vi "MainPannelFastEnabled.vi"() -> ()   [LabVIEW 2020]
uses:
  Digi/Controls/DigiMachineStates.ctl
  Digi/Digitizer_StatesMain.ctl
  <vilib>/userdefined/High Color/nirio_resource_hc.ctl
  Stage/New/StageOptions.ctl
  FileStore/Data Save State.ctl
  Gen/Generator_States.ctl
  <vilib>/Heliosphere Research LLC/Advanced Plotting Toolkit/properties/Colormap_Map.ctl
  <vilib>/Native 3D Graph/xcontrol/3DPC_SurfacePlot.xctl
  WaveClusterPacket.ctl
  ThorLabs/SubViForControl/Z Axis States.ctl
  <vilib>/UPVI/lvhdf5/library.llb/HDF5 Ref.ctl
  ImageCluster.ctl
  ThorLabs/SubViForControl/Thor_KCubeServoDCRef.ctl
  ThorLabs/SubViForControl/Thor_DeviceRef.ctl
  LongShotStates.ctl
  <vilib>/Platform/TimedLoop/XDataNode/timing_clust.ctl
  <vilib>/Platform/TimedLoop/XDataNode/nitl_modes.ctl
  <vilib>/Platform/TimedLoop/XDataNode/wakeup.ctl
  Stage/New/SettingCtrlOptions.ctl
  Stage/New/PosCtrlOptions.ctl
  Digi/Controls/FPGA VI Reference.ctl
  <extravilib>/ChannelInstances/Tag-bool/Read With Abort.vi
  <extravilib>/ChannelInstances/Tag-a[.](dbl)/Read With Abort.vi
  <extravilib>/ChannelInstances/Tag-a[.](dbl)/Write With Abort.vi
  <extravilib>/ChannelInstances/Tag-bool/Write With Abort.vi
  <extravilib>/ChannelInstances/Tag-bool/Instantiate.vi
  <extravilib>/ChannelInstances/Tag-bool/EndpointRead.vi
  <vilib>/FPGAPlugInAG/PXIe-7962R/niLvFpga_Open_PXIe-7962R.vi
  <vilib>/rvi/interface/common/dynamic/niFpgaDynamicAddResources.vi
  <vilib>/FPGAPlugInAG/Dynamic/niLvFpga_Close_Dynamic.vi
  <extravilib>/ChannelInstances/Tag-bool/Endpoint.vi
  <extravilib>/ChannelInstances/Tag-a[.](dbl)/Instantiate.vi
  <extravilib>/ChannelInstances/Tag-a[.](dbl)/EndpointRead.vi
  <extravilib>/ChannelInstances/Tag-a[.](dbl)/Endpoint.vi
  <vilib>/Platform/TimedLoop/XDataNode/XDataNode.xnode
  <vilib>/rvi/interface/nirviOpenFPGA/nirviOpenFPGA.xnode
  FPGA Bitfiles/DigitizerFPGACode(Fully_Functional)_v3.lvbitx
  <vilib>/rvi/interface/nirviCloseFPGA/nirviCloseFPGA.xnode
  <instrlib>/_niInstr/Basic Elements/v1/FPGA/niInstr Basic Elements v1 FPGA.lvlib
  <vilib>/Platform/TimedLoop/XDataNode/XDNodeRunTimeDep.lvlib
  Stage/libximc.lvlib
  <extravilib>/ChannelInstances/Tag-bool.lvlib
  <extravilib>/ChannelInstances/Tag-a[.](dbl).lvlib
  E:/Norway Project/All Hardware/New Microscope/LabVIEW/ThorLabs/Thorlabs.MotionControl.Controls.dll
  ThorLabs/Thorlabs.MotionControl.Controls.dll
  E:/Norway Project/All Hardware/New Microscope/LabVIEW/ThorLabs/ThorLabs.MotionControl.KCube.DCServoCLI.dll
  ThorLabs/ThorLabs.MotionControl.KCube.DCServoCLI.dll
  <vilib>/Heliosphere Research LLC/Advanced Plotting Toolkit/Advanced Plotting Toolkit.lvlib
panel:
  out "ProgressBar\nLongShot":u8(slide) scale=0.0..100.0
  in  "Long Shot Time (us)":dbl
  in  "LongShot":bool
  out "At Limit":bool
  out "Z Moving?":bool
  in  "Z_Speed (mm/s)":dbl=0.5 caption="Speed (mm/s)" min=0.0 max=10.0 step=0.1
  out "Z Open?":bool
  out "Z (mm)":dbl format="%#.3g"
  in  "Z_Stop":bool
  in  "Z_MoveDown":bool
  in  "Z_Move Up":bool
  in  "Z Step (mm)":dbl=0.1 min=0.0 max=50.0 step=0.01
  out "RemainingTimeString":string
  out "ProgressBar":u8(slide) scale=0.0..100.0
  out "Image Display":dbl[][](graph)
  in  "Colormap Selector":T1(ring)=enum."gray"
  in  "Save Img":bool
  in  "LogMode":bool
  in  "Start Digitizer UI Bttn":bool
  out "Max Index (s)":dbl format="%#_3p"
  out "Max Val (V)":dbl format="%#_3p"
  in  "Delay_Scroll_Range":dbl=2.0 caption="Range"
  in  "FineDelayControl":dbl(slide)=1.0 step=0.1 scale=19.5..23.5
  in  "Amplitude Range":cluster{"Slider 1":dbl, "Slider 1":dbl}(slide)={"Slider 1"=1.0, "Slider 1"=1.6299559471365639} scale=-2.5..2.5
  in  "Pause Triggger":bool caption="Pause"
  in  "Delay(us)":sgl min=0 step=0.1 format="%#_4p"
  in  "Time Division":u8(slide)=1 max=2 step=1 scale=0.0..2.0
  in  "Amplitude \nAveraging":u16(slide)=1 caption="Amplitude Averaging" scale=0.0..7.0 scale format="%#.2g"
  in  "Record Size":u16=1024
  in  "RIO Resource":T2="PXI1Slot2"
  out "Configured?":bool
  out "TIS Configured?":bool
  out "Range (Vpp)":dbl=1.3
  out "Digitizer On":bool
  out "Waveform [LIVE]":cluster{"Start Time":dbl, dbl, ext[]}(graph)
  in  "TriggerDigi":bool
  in  "Scanning":bool
  in  "Single Shot":bool
  in  "LIVE":bool
  in  "Transducer Freq (Hz)":u64
  in  "Temperature (C)":dbl
  in  "Remarks":string
  in  "Immersion Medium":string
  in  "EXIT APP":bool
  in  "Save to File":bool=TRUE caption="Checkbox"
  out "No Trig Miss":bool
  in  "FileName":string="testing"
  in  "File Store Directory":path=path "C:/Prakhar/ScratchStart/Labview16/TrashTest"
  out "File Open?":bool
  out "X Step Size (R)":sgl format="%#_2g"
  out "Y Step Size (R)":sgl format="%#_2g"
  out "Scan Time (Approx.)":string
  out "Total Pixels":u64
  out "Moving?":bool
  out "Stage Position":cluster{sgl[], sgl[]}(graph) caption="XY Graph - Dark"
  in  "X Position Abs":dbl caption="X Position"
  in  "Y Position Abs":dbl caption="Y Position"
  out "Line Count":u64=6 caption="Y Pixels"
  out "Pixel Count":u64=6 caption="X Pixels"
  in  "X Start":sgl
  in  "X End":sgl=10.0
  in  "Y Start":sgl
  in  "Y End":sgl=8.0
  in  "Y Step Size":sgl=0.5
  in  "X Step Size":sgl=0.5
  in  "Scan Mode":enum16{"Raster", "Serpentine"}(ring)
  in  "Speed Control (mm/s)":sgl(slide)=4.0 min=0.1 scale=0.1..5.0
  in  "AbsMove":bool
  in  "Outline":bool
  in  "Start Stage":bool
  in  "Stop Motion":bool
  in  "Zero":bool
  in  "Right":bool
  in  "Left":bool
  in  "Move to Start":bool
  in  "Down":bool
  in  "Up":bool
  out "X Position":dbl format="%#.3g"
  out "Y Position":dbl format="%#.3g"
  in  "Move Step":dbl=1.0
  in  "Stop Stage":bool
  out "Controller Open?":bool
  in  "Developer Options Control":T3(tab)
  in  "Stop Gen App":bool
  out "Gen State":T4
  out "Error Out Gen":errorcluster
  in  "Send vi Trig":bool
  out "Gain":dbl
  out "Offset Factor":dbl
  out "Amplitudes":dbl[](array[numeric]) format="%.2f"
  out "Sampling Frequency (Hz)":u64
  out "Waves per Pixel":u32
  in  "Ext/nViTrig":bool=TRUE
  in  "Machine Mode":T5(ring)=enum."Normal"
  in  "Stop Stage App":bool
  out "Error Out Stage":errorcluster
  in  "Next Coordinate Index":i32
  in  "EdgePt/nPixelMap":bool=TRUE
  out "Coordinate Array":sgl[][](array[numeric])
  out "Step Sizes":sgl[](array[numeric])
  out "Peripheral Coordis":sgl[][](array[numeric])=[[0.0, 0.0], [1.8, 0.0], [3.6, 0.0], [5.3999996, 0.0], [7.2, 0.0], [9.0, 0.0], [9.0, 2.0], [7.2, 2.0], [5.3999996, 2.0], [3.6, 2.0], [1.8, 2.0], [0.0, 2.0], [0.0, 4.0], [1.8, 4.0], [3.6, 4.0], [5.3999996, 4.0], [7.2, 4.0], [9.0, 4.0], [9.0, 6.0], [7.2, 6.0], [5.3999996, 6.0], [3.6, 6.0], [1.8, 6.0], [0.0, 6.0], [0.0, 8.0], [1.8, 8.0], [3.6, 8.0], [5.3999996, 8.0], [7.2, 8.0], [9.0, 8.0], [9.0, 10.0], [7.2, 10.0], [5.3999996, 10.0], [3.6, 10.0], [1.8, 10.0], [0.0, 10.0]]
  in  "Correction Table Path (Hidden)":path
  out "Serial nos":u32[](array[numeric])
  out "Calibration":cluster{dbl, "MicrostepMode":u32}[](array[cluster])
  out "IDs":i32[](array[numeric])
  in  "X Max Stage":dbl=220.0 format="%#_13g"
  in  "Y Maximum":dbl=220.0
  out "Stage Status":T6
  out "Z Axis State":T7
  out "Wave Count Zero":bool
  in  "CountReset":bool
  in  "Trigger Digi Single":bool
  in  "Start Digi":bool
  in  "Stop Digi App":bool caption="Stop Digi \nApplication"
  in  "Digi Machine Mode":T8=enum."Single Shot Mode"
  out "Waves Count":u64
  in  "Imaging":bool
  out "Digi State":T9
  out "nDigiLoopRunning":bool
  out "error out Digi":errorcluster
  out "Wave out packet":T10
  out "Error Out FileIO":errorcluster
  in  "Done Recording":bool
  in  "Record Data":bool
  in  "Open File":bool
  in  "Stop File App":bool
  out "FileStore State":T11
  out "Scan Running":bool=TRUE
  out "Scan Complete":bool=TRUE
  out "AmplitudeArray":dbl[](array[numeric])
  out "IndexArray":dbl[](array[numeric])
  in  "Map":T12
  in  "ColorBar":bool
  in  "Axis":bool
  out "Scanned Image":picture
  out "Topography Plot":refnum<class "Base Datatype.lvclass">[](xcontrol)
  out "LongShotRunTimes":u32=6
  out "FilenameSimeStamped":string
  out "FileDirectoryFinal":path
  out "total time (sec)":sgl
  in  "Generator  Port":refnum<k15>="PXI1Slot3"
  out "Actual Sample Rate":dbl format="%#_6p"
  in  "Use Default Wave Settings":bool=TRUE caption="Checkbox"
  in  "Start Gen":bool
  in  "stop Gen":bool
  out "Generator On":bool
  out "Input Waveform":dbl[](graph)
  # "SAVE ALL CONFIGS TO FILE AND LOAD IT"
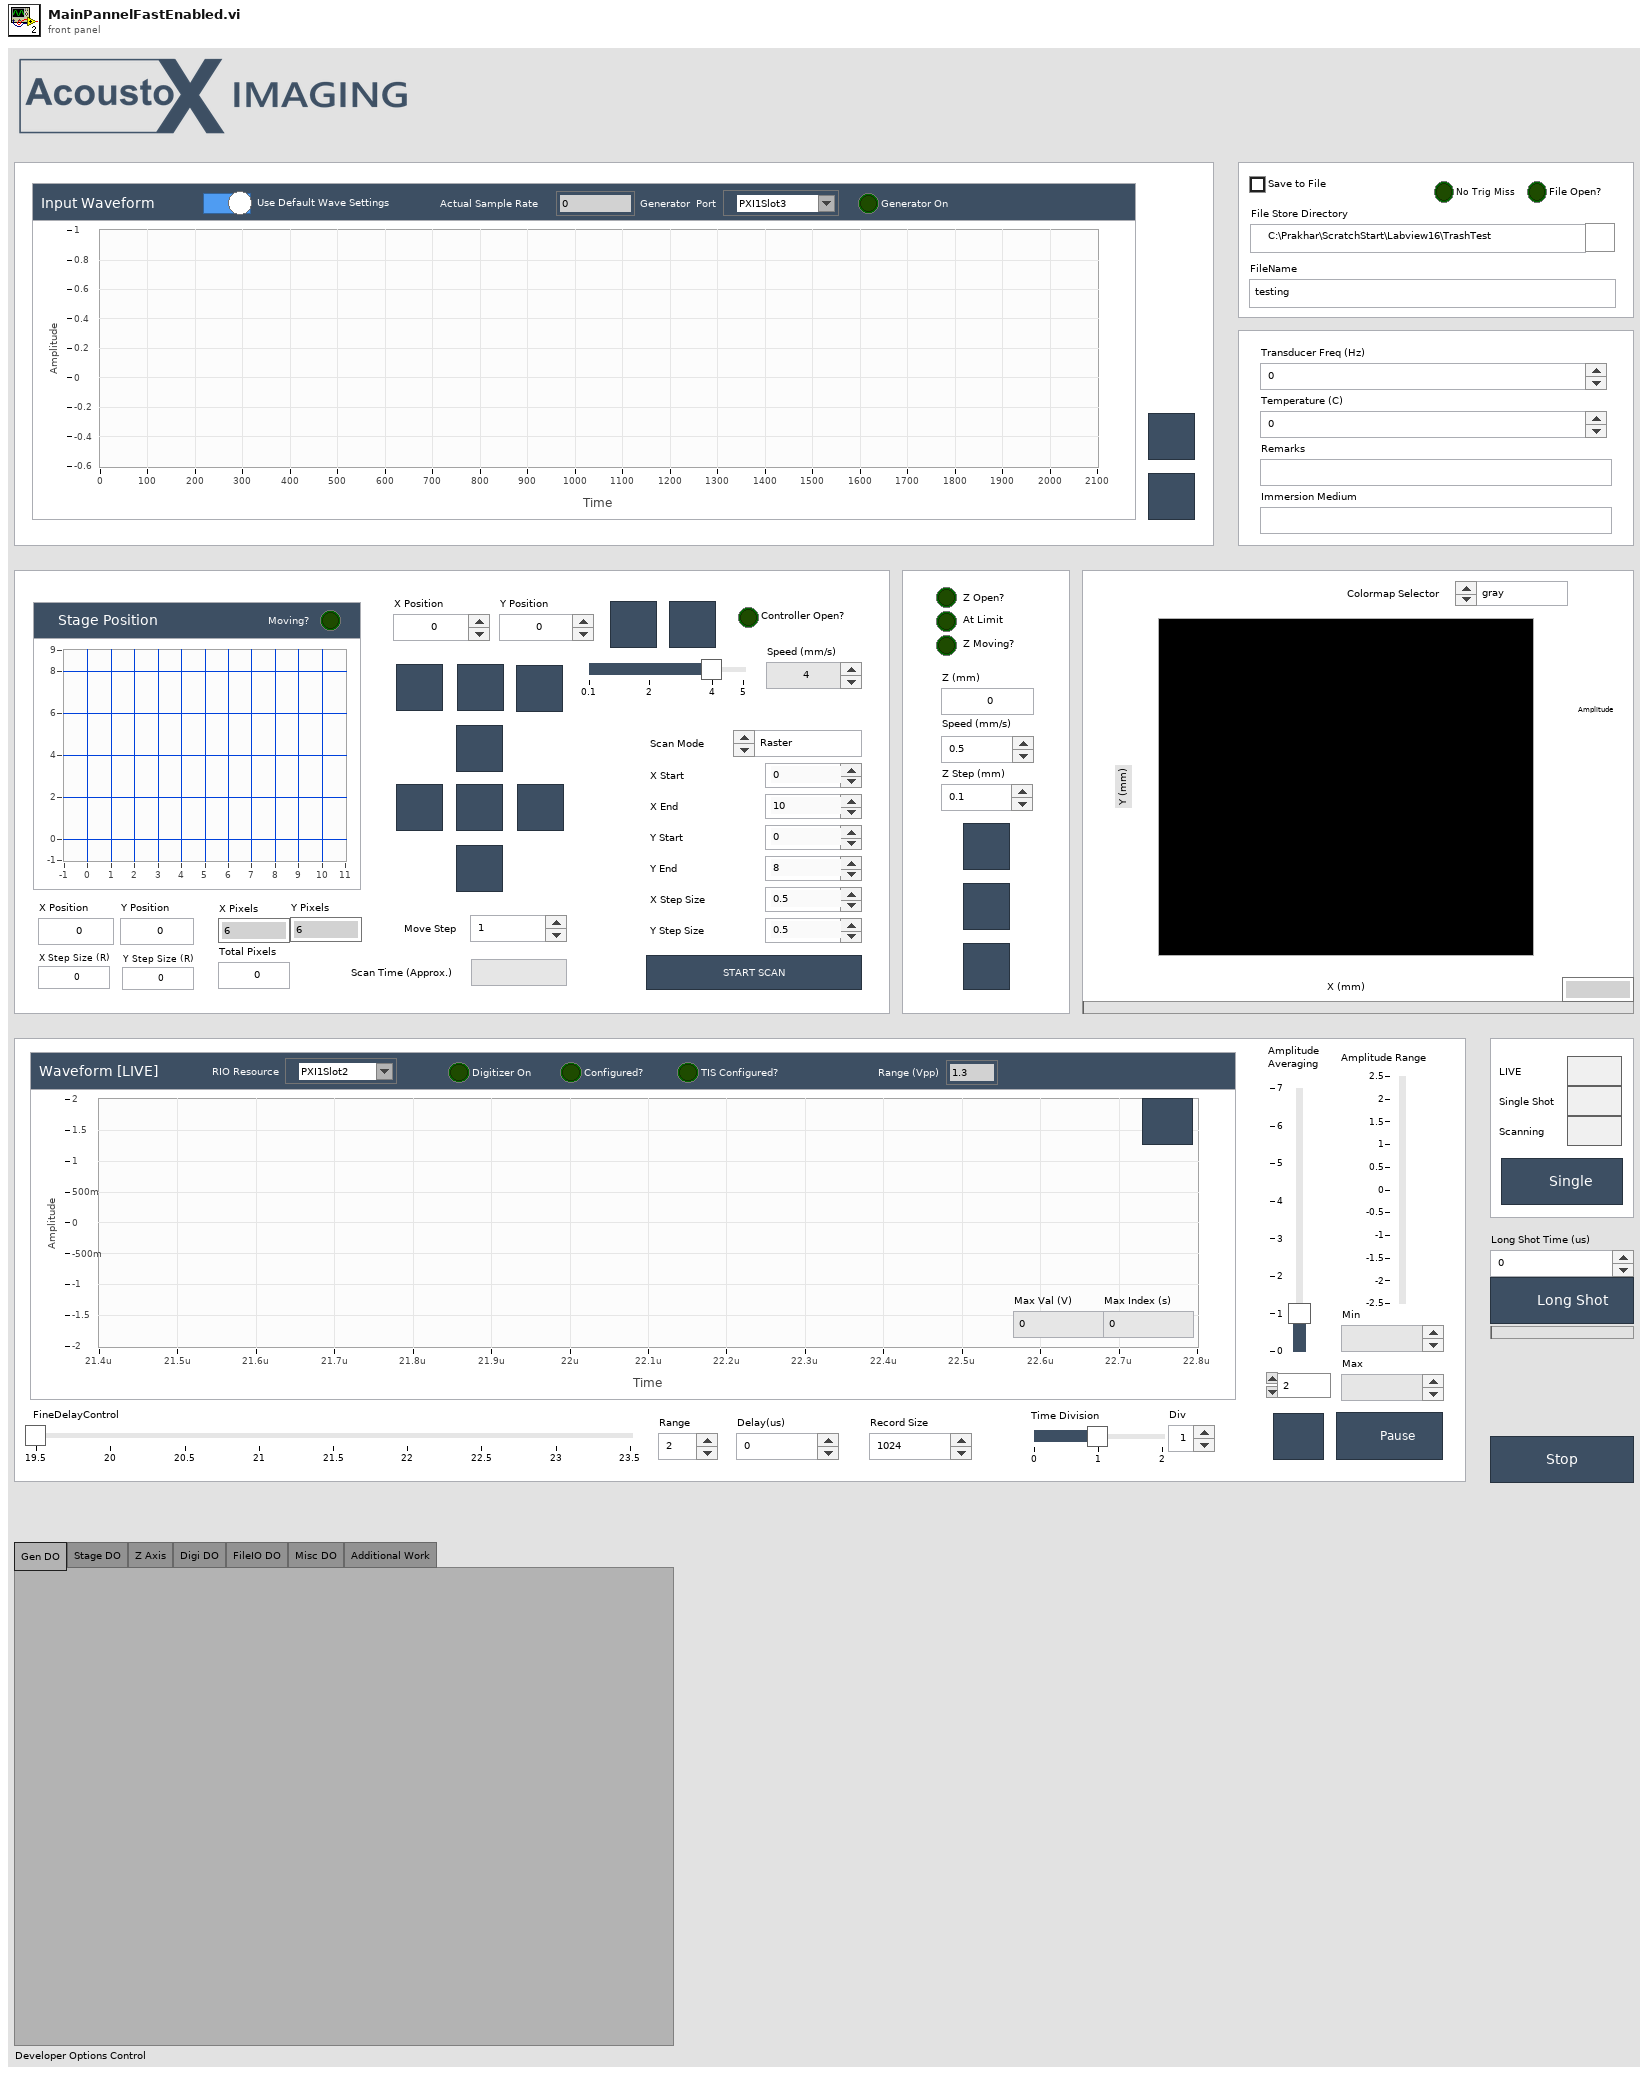
[diagram p1: front panel]
types:
  T1 = enum16{"fire", "rainbow", "gray", "inverse gray", "ice", "original"}
  T2 = typedef "nirio_resource_hc.ctl" = tag
  T3 = enum32{"Gen DO", "Stage DO", "Z Axis", "Digi DO", "FileIO DO", "Misc DO", "Additional Work"}
  T4 = typedef "Generator_States.ctl" = enum16{"Idle", "GenerateWaveArray", "InitGen", "SendVITrig", "CloseGen", "CloseApp"}
  T5 = enum16{"Scanning Mode", "Perimeter Mode", "Normal"}
  T6 = typedef "StageOptions.ctl" = enum16{"Idle", "Init", "Set Speed", "GenerateMotionPoints", "Scan_Start", "Scan_MoveNext", "Scan_SyncSet", "Scan_Get Pos", "Scan_Complete", "Cmd_MoveAbs", "Cmd_CloseControllers", "Cmd_MoveUp", "Cmd_MoveDown", "Cmd_MoveLeft", "Cmd_MoveRight", "Cmd_MoveStart", "Cmd_MoveZero", "Cmd_GetPos", "Cmd_Stop", "Sync_On", "Sync_Off", "Stop Motion", "CloseApplication"}
  T7 = typedef "Z Axis States.ctl" = enum16{"Idle", "Init", "cmd_MoveUp Rel", "cmd_MoveDown Rel", "cmd_GetPos", "cmd_SetVel", "cmd_stop", "Close Z"}
  T8 = typedef "DigiMachineStates.ctl" = enum16{"Scanning Mode", "Live Mode", "Single Shot Mode", "Idle Mode"}
  T9 = typedef "Digitizer_StatesMain.ctl" = enum16{"Idle", "Init", "SetParam", "VITrig", "Read", "CloseDigi", "CloseApp"}
  T10 = typedef "WaveClusterPacket.ctl" = cluster{"Wave Count":u64, "Wave":i16[]}
  T11 = typedef "Data Save State.ctl" = enum16{"Idle", "Open File", "Write Attributes", "Append Data", "Close File", "Close App"}
  T12 = typedef "Advanced Plotting Toolkit.lvlib/Colormap_Map.ctl" = enum16{"Automatic", "Rainbow", "Hot and Cold", "White-Black", "White-Blue", "White-Green", "White-Red", "Fire", "Water", "Earth", "Air", "Pastel", "Banded", "Stepped"}
  T13 = typedef "LongShotStates.ctl" = enum16{"Idle", "Start Gen", "Set Digi Mode", "Clear Wave Count", "Set Initial Param", "Set Param", "Take Shot", "UpdateParam", "Show Data"}
  T14 = typedef "Thor_DeviceRef.ctl" = refnum<k24>
  T15 = typedef "Thor_KCubeServoDCRef.ctl" = refnum<k24>
  T16 = typedef "ImageCluster.ctl" = cluster{"Wave Count":u64, "Amplitude":i16, "Index":u16}
  T17 = typedef "HDF5 Ref.ctl" = refnum<k1>
  T18 = typedef "XDNodeRunTimeDep.lvlib/timing_clust.ctl" = cluster{"Expected End [f-1]":u64, "Actual End [f-1]":u64, "Finished Late? [f-1]":bool, "Expected End [i-1]":u64, "Actual End [i-1]":u64, "Finished Late? [i-1]":bool, "Expected Start [i]":u64, "Actual Start [i]":u64, "Expected Start [f]":u64, "Actual Start [f]":u64, "Source Name":string, "Structure Name":string, "Period":i64, "Deadline":i64, "Offset":i64, "Start":i64, "Priority":i32, "Timeout":i32, "Mode":T19, "Wakeup Reason":T20, "Error":errorcluster, "Source Type":string, "Secondary Source Type":string, "Global End Time":u64, "Global Start Time":u64, "Frame Duration":u64, "Iteration Duration":u64, "Assigned CPU":i32, "I/O Scan Engine Mode":u32}
  T19 = typedef "XDNodeRunTimeDep.lvlib/nitl_modes.ctl" = enum32{"No Change", "Process missed periods, maintain original phase", "Discard missed periods, maintain original phase", "Process missed periods, ignore original phase", "Discard missed periods, ignore original phase"}
  T20 = typedef "XDNodeRunTimeDep.lvlib/wakeup.ctl" = enum32{"Normal", "Aborted", "Asynchronous wakeup", "Timing source error", "Timed loop error", "Timeout"}
  T21 = typedef "SettingCtrlOptions.ctl" = enum16{"Set X", "Set Y", "Set X and Y", "Get Settings", "None"}
  T22 = typedef "PosCtrlOptions.ctl" = enum16{"Move X", "Move Y", "Both X and Y", "Read Pos", "None"}
  T23 = typedef "Tag-a[.](dbl).lvlib/))Channel.ctl" = refnum<queue>
  T24 = typedef "FPGA VI Reference.ctl" = refnum<k20>
  T25 = typedef "imagedata.ctl" = cluster{"image type":i32, "image depth":i32, "image":u8[], "mask":u8[], "colors":u32[], "Rectangle":cluster{"left":i16, "top":i16, "right":i16, "bottom":i16}}
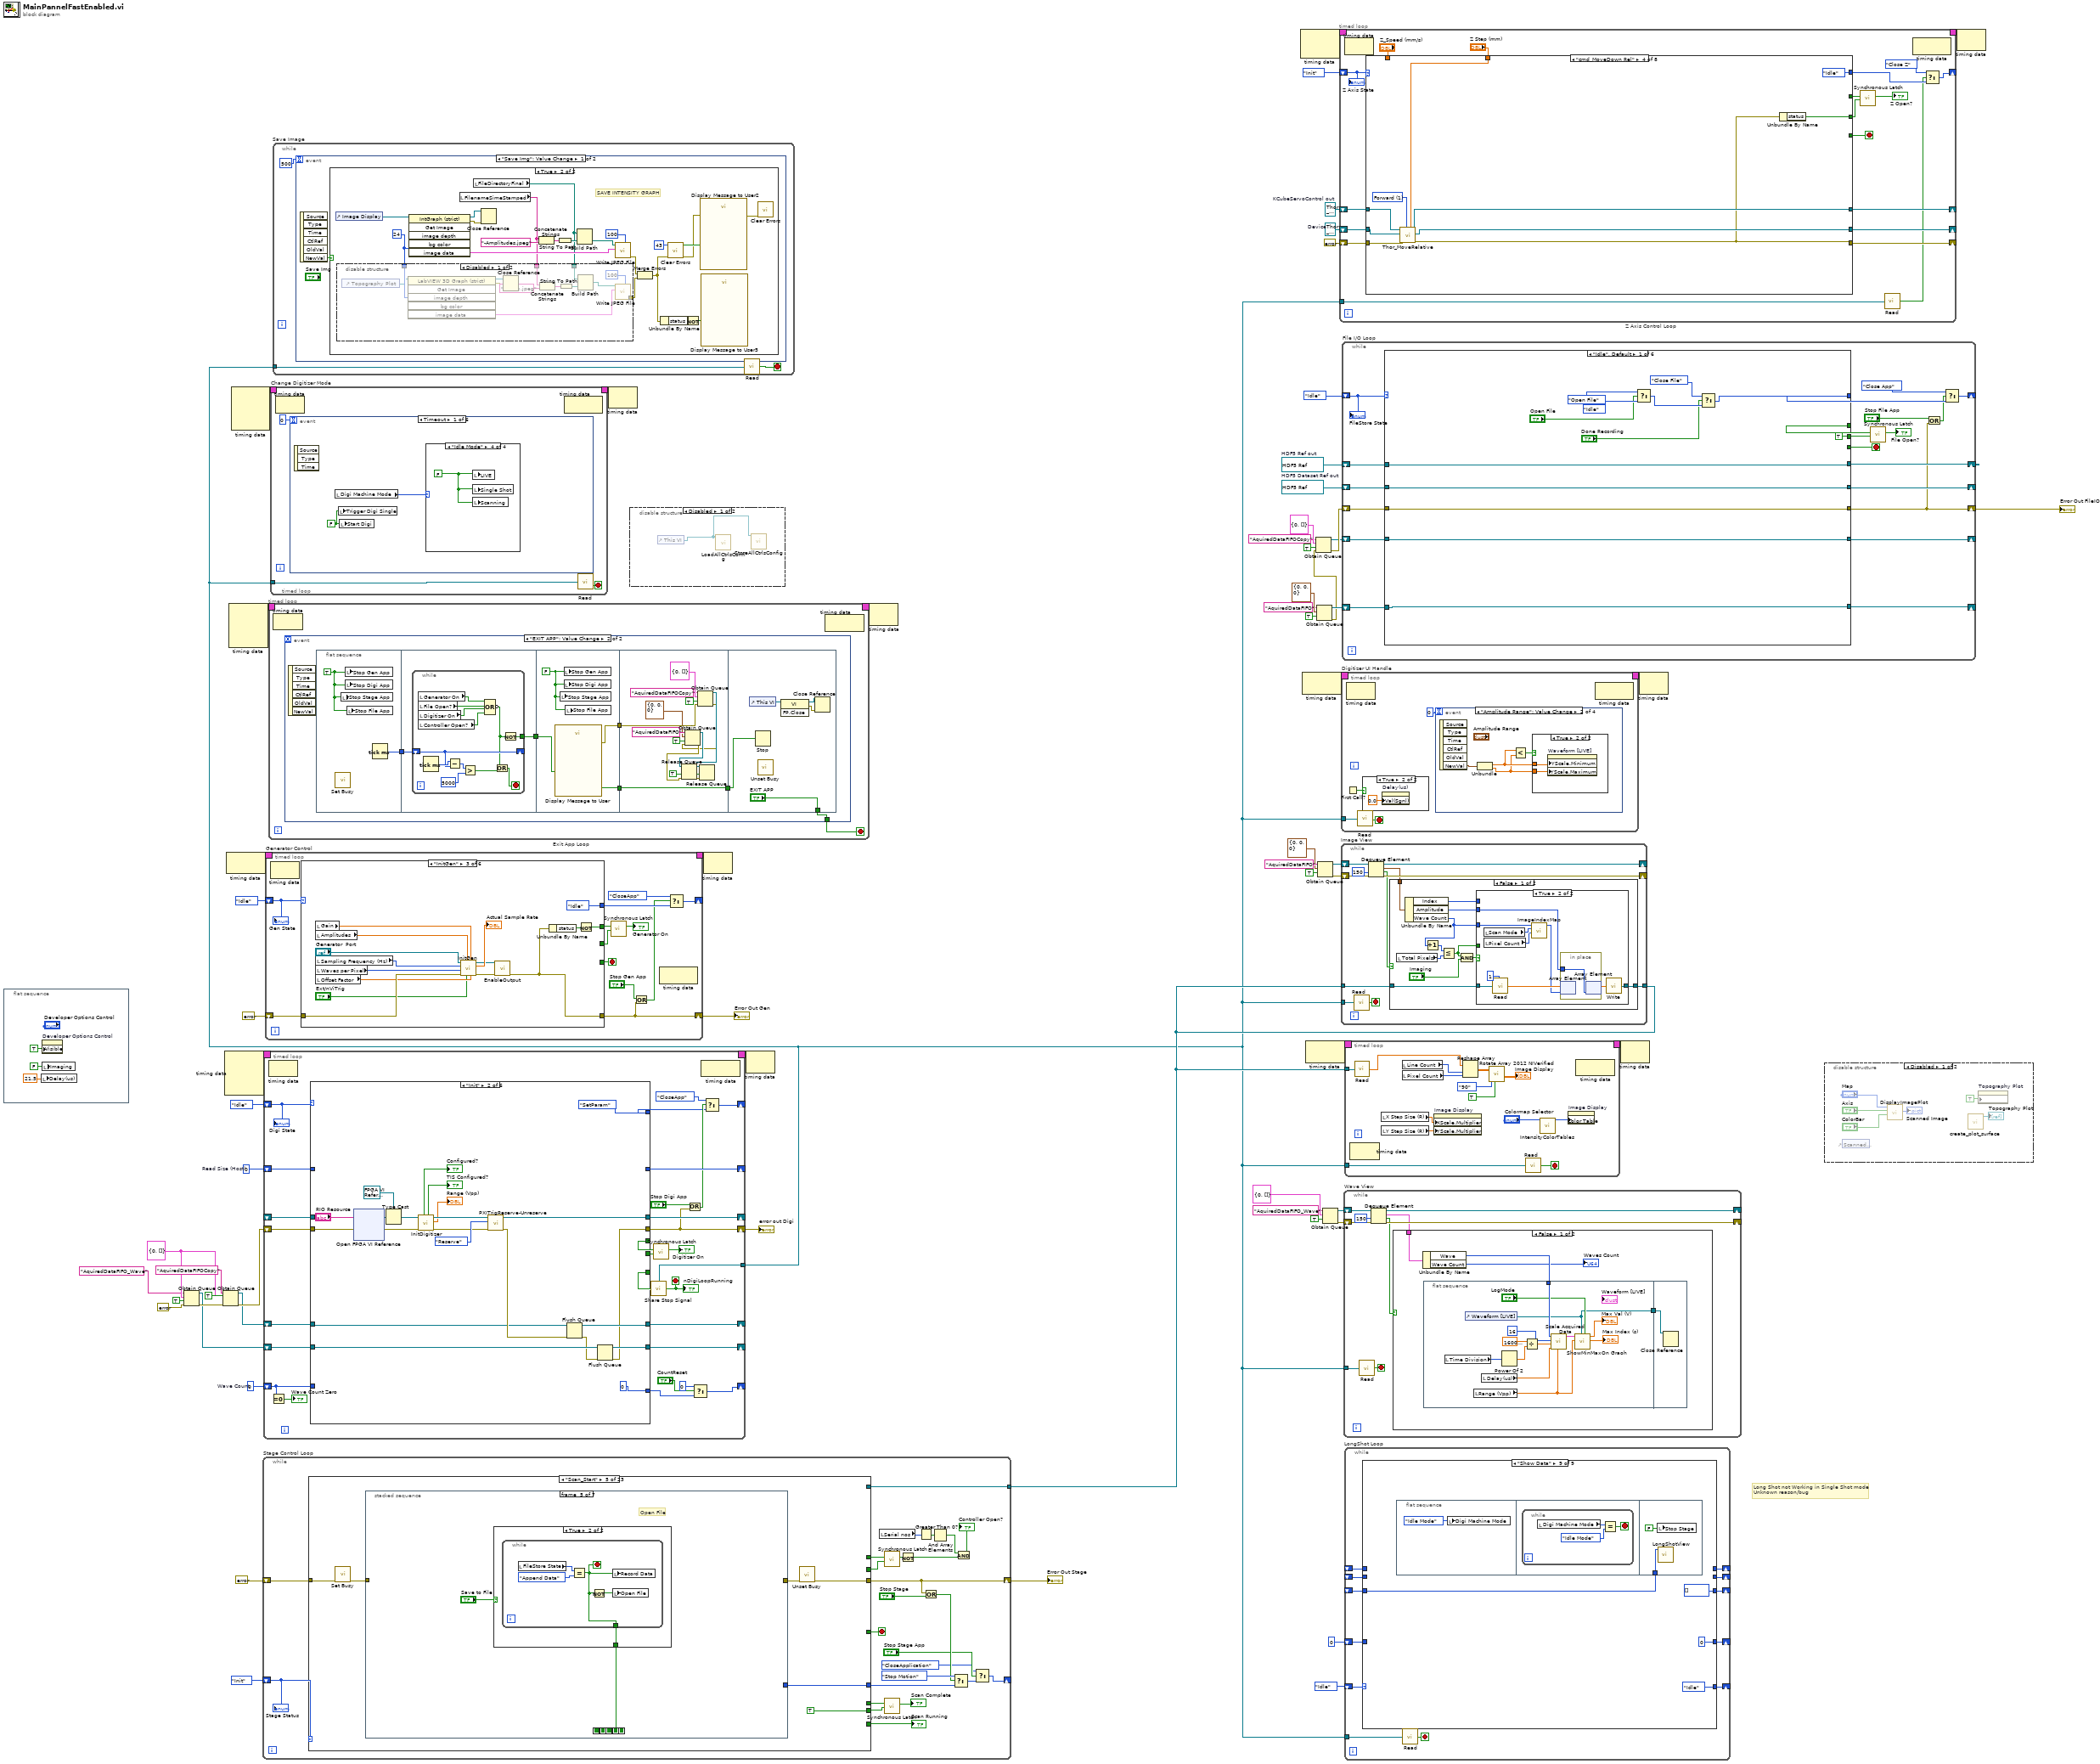
[diagram p0: block diagram]
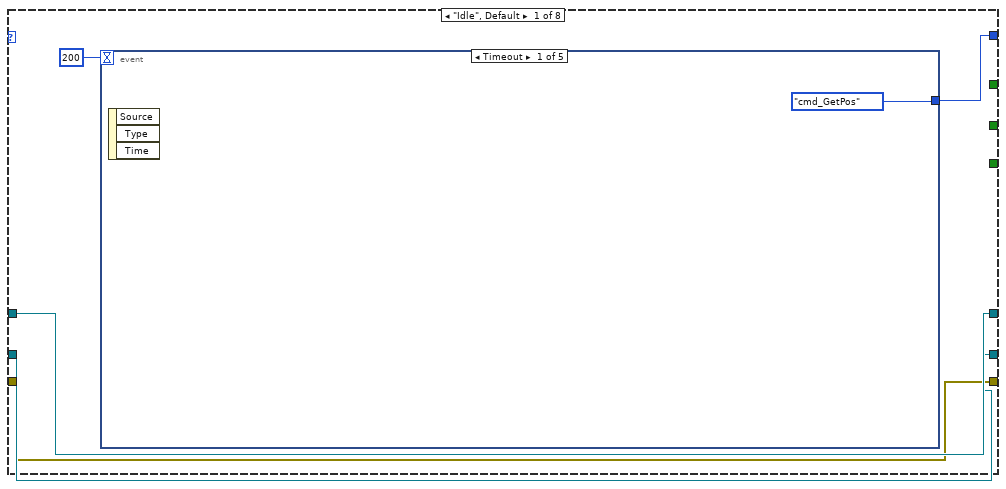
[diagram p2: hidden frame]
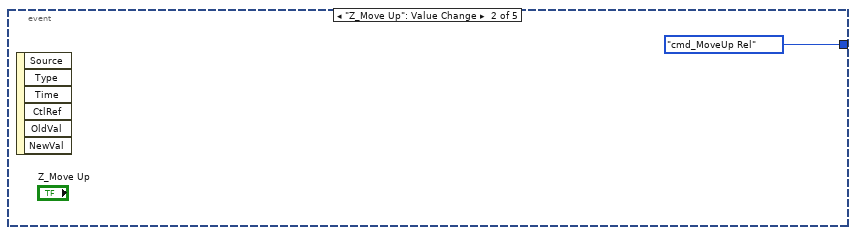
[diagram p3: hidden frame]
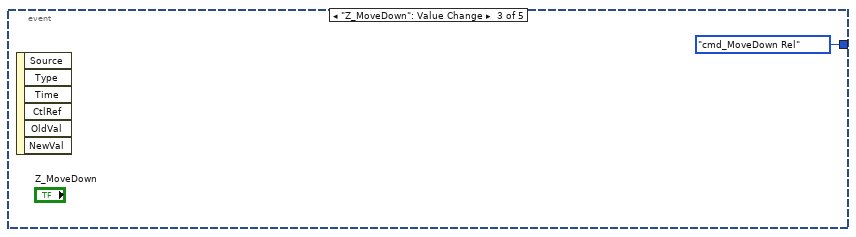
[diagram p4: hidden frame]
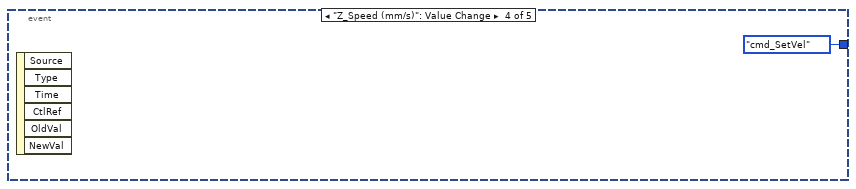
[diagram p5: hidden frame]
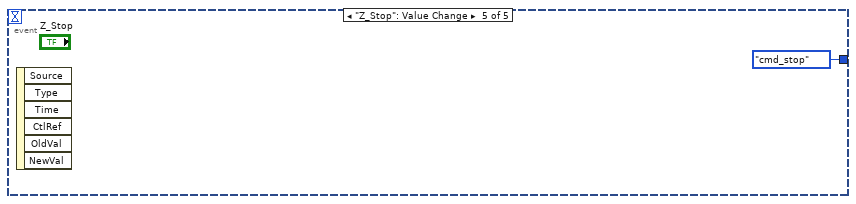
[diagram p6: hidden frame]
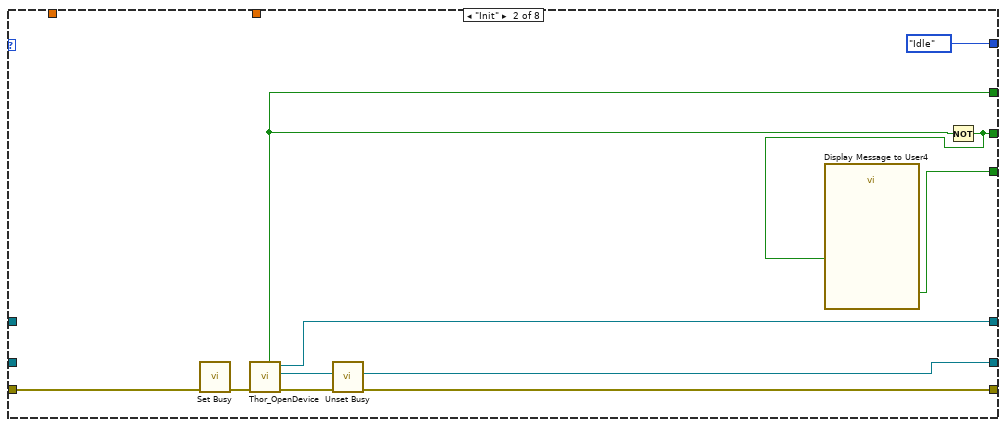
[diagram p7: hidden frame]
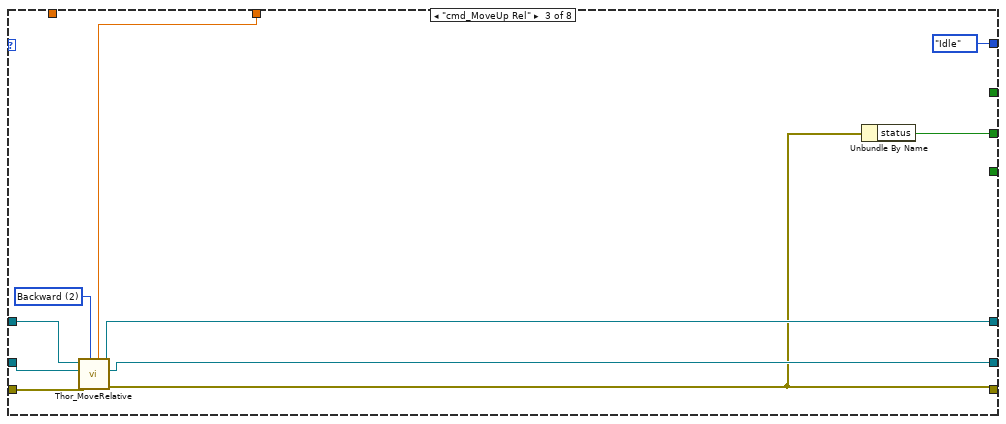
[diagram p8: hidden frame]
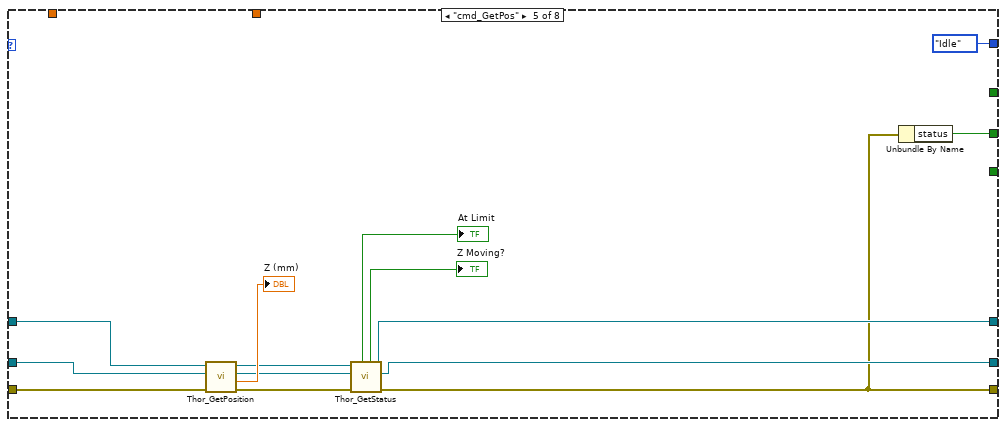
[diagram p9: hidden frame]
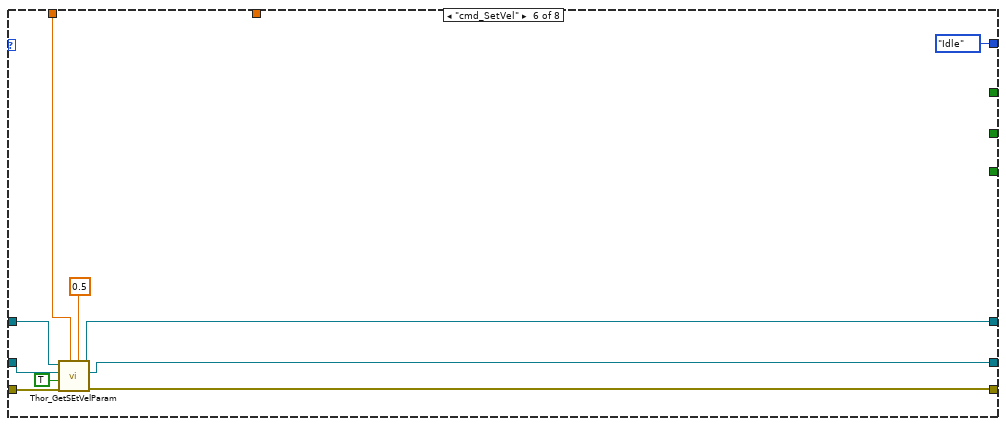
[diagram p10: hidden frame]
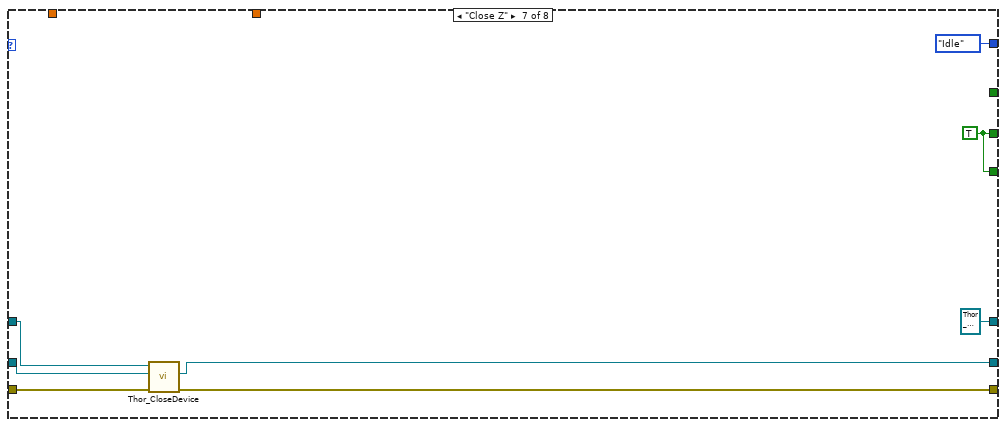
[diagram p11: hidden frame]
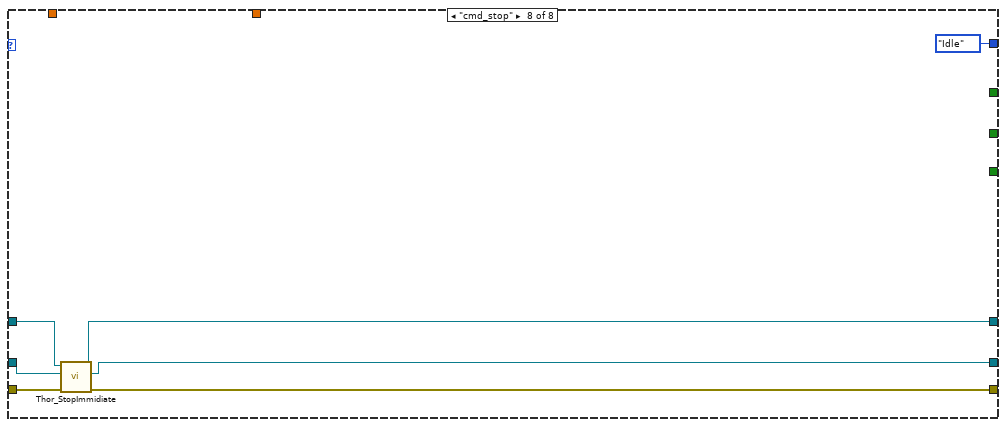
[diagram p12: hidden frame]
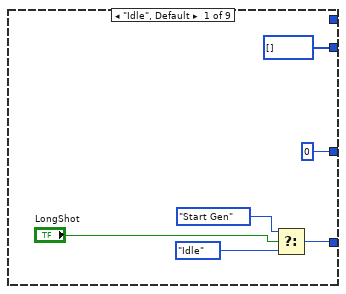
[diagram p13: hidden frame]
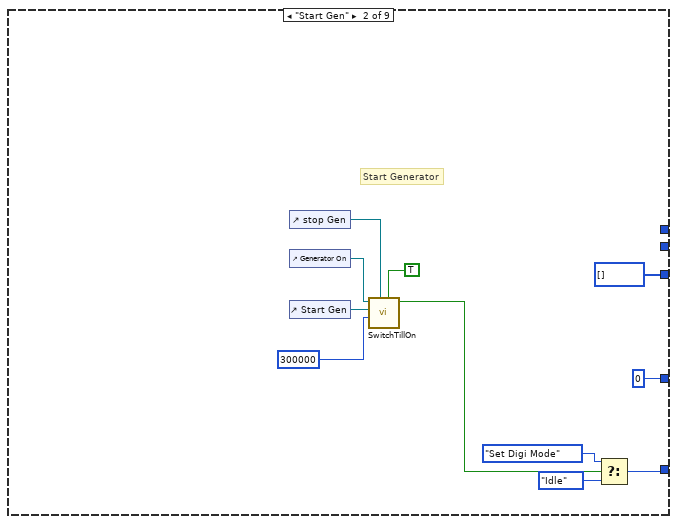
[diagram p14: hidden frame]
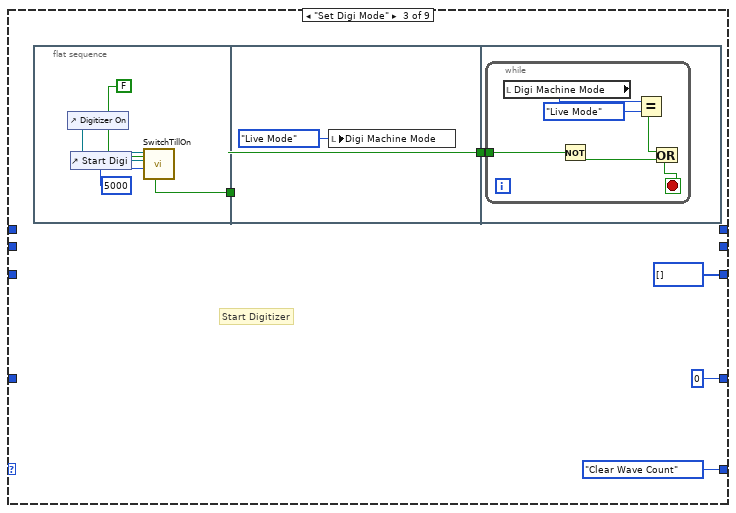
[diagram p15: hidden frame]
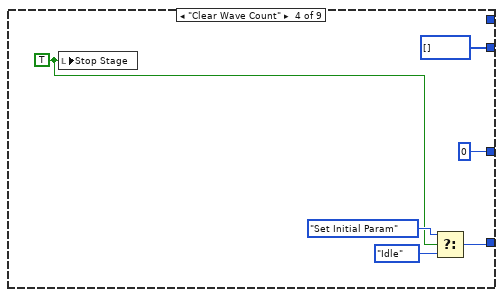
[diagram p16: hidden frame]
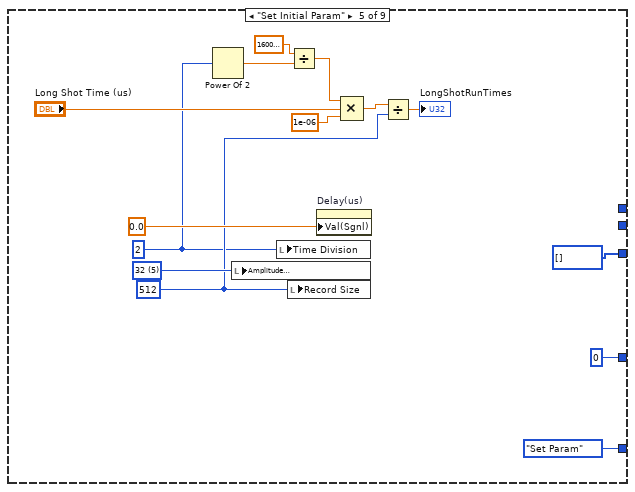
[diagram p17: hidden frame]
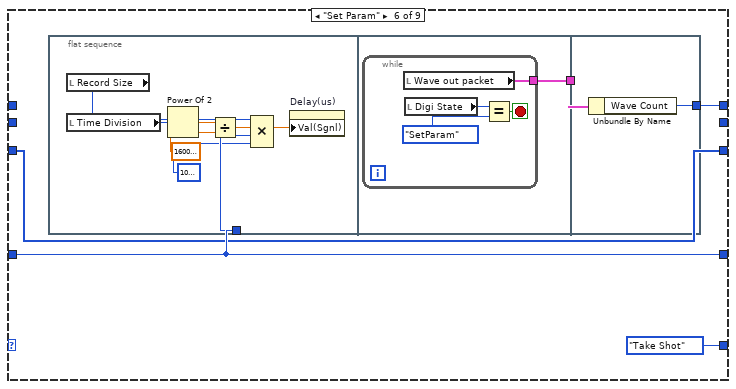
[diagram p18: hidden frame]
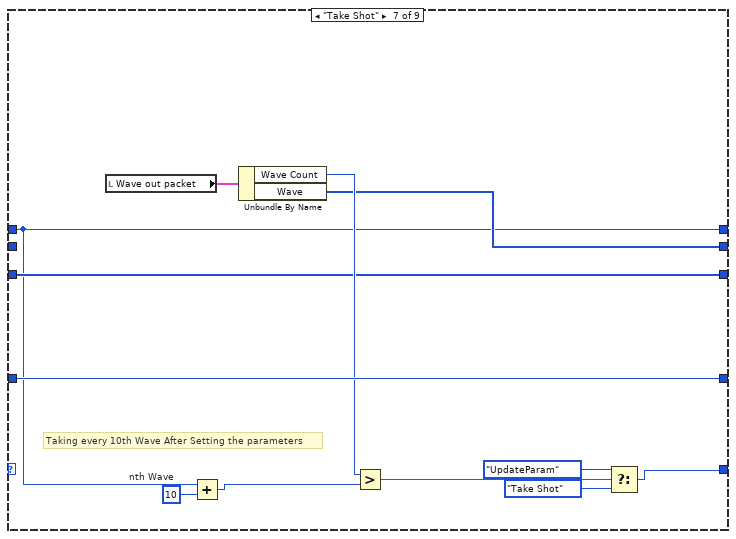
[diagram p19: hidden frame]
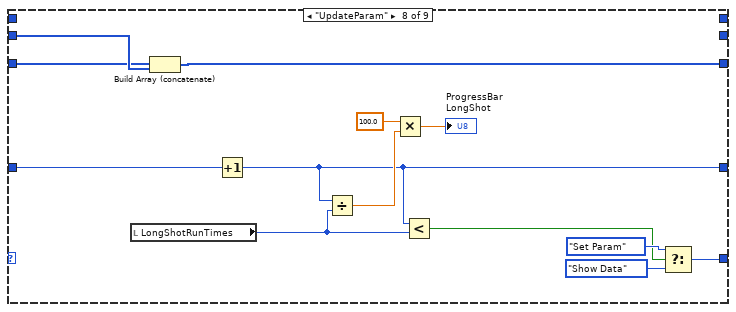
[diagram p20: hidden frame]
diagram:
  w6 = T14 refnum  # Device
  w7 = T15 refnum  # KCubeServoControl out
  w44 = u64 0  # Wave Count
  w31 = T10 {"Wave Count"=0, "Wave"=[]} ("input cluster")
  w50 = T17 refnum items=["HDF5 Ref"]  # HDF5 Dataset Ref out
  w51 = T17 refnum items=["HDF5 Ref"]  # HDF5 Ref out
  w61 = u16 0  # Read Size (Host)
  # "Long Shot not Working in Single Shot mode\nUnknown reason/bug"
  n1 = flat-sequence {
    frame #0 {
      n2 = local write "Delay(us)"(sgl 21.5 ("Delay(us)")) -> ()
      n3 = property on="Developer Options Control" class="TabCtl (strict)"("Visible"=TRUE) -> ()  [unwired: 2 in, 2 out]
      n4 = local write "Imaging"(FALSE ("Imaging")) -> ()
    }
  }
  n5 = Obtain Queue(name (unnamed)="AquiredDataFIFO_Wave", element data type=w31, create if not found? (T)=TRUE, error in (no error)=errorcluster {"status"=FALSE, "code"=0, "source"=""}) -> (queue out=w32:refnum<queue>, error out=w35:errorcluster)  [unwired: 1 in, 1 out]
  n6 = Obtain Queue(name (unnamed)="AquiredDataFIFOCopy", element data type=w31, create if not found? (T)=TRUE, error in (no error)=w35) -> (queue out=w46:refnum<queue>, error out=w47:errorcluster)  [unwired: 1 in, 1 out]
  n7 = node-c288() -> (w16:T18)  [unwired: 4 in]
  n8 = node-c288() -> (w58:T18)  [unwired: 1 in]
  n9 = node-c288() -> (w11:T18)  [unwired: 4 in]
  n10 = node-c288() -> (w37:T18)  [unwired: 4 in]
  n11 = while "Stage Control Loop" {
    shift-right: [w83] -> _
    shift-left: StageOptions."Init" -> [w94]
    shift-right: [w91] -> w24
    shift-left: errorcluster {"status"=FALSE, "code"=0, "source"=""} ("error out") -> [w92]
    tunnel: [w70] -> w12
    stop <- w84 stop-if-true
    n12 = case shown="\"Scan_Start\"" w94 {
      tunnel: [w99 w195 w218 w257 w262 w392 w407 w421 w461 w483 w492 w499 w510 w520 w530 w539 w547 w562 w568 w579 w588 w596 w607] -> w91
      tunnel: w92 -> [w99 w193 w219 w256 w264 w393 w408 w422 w459 w484 w493 w498 w511 w521 w531 w540 w548 w563 w567 w580 w589 w595 w606]
      tunnel: [w98 StageOptions."Set Speed" StageOptions."GenerateMotionPoints" w241 w265 w383 StageOptions."Scan_MoveNext" w418 StageOptions."Idle" StageOptions."Idle" StageOptions."Idle" StageOptions."Idle" StageOptions."Idle" StageOptions."Idle" StageOptions."Idle" StageOptions."Idle" StageOptions."Idle" StageOptions."Idle" StageOptions."Idle" StageOptions."Idle" StageOptions."Idle" StageOptions."Idle" StageOptions."Idle"] -> w89
      tunnel: [_ _ _ _ _ _ _ _ _ _ _ _ _ _ _ _ _ _ _ _ _ w592 w602] -> w87
      tunnel: [_ w196 _ _ _ _ _ _ _ _ _ _ _ _ _ _ _ _ _ _ _ _ _] -> w85
      tunnel: [_ _ _ _ _ _ _ _ _ _ _ _ _ _ _ _ _ _ _ _ _ _ w602] -> w84
      tunnel: [_ _ _ _ _ _ _ _ TRUE ("X SyncOut Enabled") _ _ _ _ _ _ _ _ _ _ _ _ _ _] -> w74
      tunnel: [TRUE ("EdgePt/nPixelMap") TRUE ("EdgePt/nPixelMap") TRUE ("EdgePt/nPixelMap") TRUE ("EdgePt/nPixelMap") TRUE ("EdgePt/nPixelMap") _ _ _ _ _ _ _ _ _ _ _ _ _ _ _ _ _ _] -> w72
      tunnel: [_ _ _ _ _ TRUE ("Moving?") TRUE ("Moving?") w409 FALSE ("Moving?") _ _ _ _ _ _ _ _ _ _ _ _ _ _] -> w71
      tunnel: [_ _ _ w223 _ _ _ _ _ _ _ _ _ _ _ _ _ _ _ _ _ _ _] -> w70
      frame "Idle", Default {
        n13 = First Call?() -> (First Call?: T/F=w96:bool)
        n14 = event shown="[1] \"Up\": Value Change" {
          selector: _ -> [_ _ _ _ _ _ _ _ _ _ _ _ _]
          dyn-events: _ -> [_ _ _ _ _ _ _ _ _ _ _ _ _]
          timeout: 100 -> [_ _ _ _ _ _ _ _ _ _ _ _ _]
          tunnel: [w102 StageOptions."Cmd_MoveUp" StageOptions."Cmd_MoveDown" StageOptions."Cmd_MoveStart" StageOptions."Cmd_MoveLeft" StageOptions."Cmd_MoveRight" StageOptions."Cmd_MoveZero" StageOptions."Cmd_Stop" StageOptions."GenerateMotionPoints" StageOptions."GenerateMotionPoints" StageOptions."Set Speed" w174 StageOptions."Cmd_MoveAbs"] -> w98
          event Timeout {
            n15 = event-data() -> ()  [unwired: 1 in, 3 out]
            n16 = local read "Controller Open?"() -> (w103:bool)
            n17 = case shown="False" w103 {
              tunnel: [StageOptions."Init" StageOptions."Cmd_GetPos"] -> w102
              frame False {
              }
              frame True {
              }
            }
          }
          event "Up": Value Change {
            w106 = 0.0  # Y Start
            w108 = sgl 0.0  # X Start
            w111 = 1.0  # Offset
            n18 = event-data() -> ()  [unwired: 1 in, 6 out]
            n19 = local read "X Max Stage"() -> (w109:dbl)
            n20 = local read "Y Maximum"() -> (w107:dbl)
            n21 = Add(x=w111, y=w109) -> (x+y=w113:dbl)
            n22 = Subtract(x=w108, y=w111) -> (x-y=w114:dbl)
            n23 = Subtract(x=w106, y=w111) -> (x-y=w110:dbl)
            n24 = Add(x=w107, y=w111) -> (x+y=w112:dbl)
            n25 = Build Array(w108, w109) -> (w116:dbl[])
            n26 = Build Array(w106, w107) -> (w115:dbl[])
            n27 = property on="Stage Position" class="XYGraph (strict)"("XScale.Maximum"=w113, "XScale.Minimum"=w114, "YScale.Maximum"=w112, "YScale.Minimum"=w110, "XScale.MarkerVals[]"=w116, "YScale.MarkerVals[]"=w115) -> ()  [unwired: 2 in, 2 out]
          }
          event "Down": Value Change {
            w118 = 0.0  # Y Start
            w120 = sgl 0.0  # X Start
            w123 = 1.0  # Offset
            n28 = event-data() -> ()  [unwired: 1 in, 6 out]
            n29 = local read "X Max Stage"() -> (w121:dbl)
            n30 = local read "Y Maximum"() -> (w119:dbl)
            n31 = Add(x=w123, y=w121) -> (x+y=w125:dbl)
            n32 = Subtract(x=w120, y=w123) -> (x-y=w126:dbl)
            n33 = Subtract(x=w118, y=w123) -> (x-y=w122:dbl)
            n34 = Add(x=w119, y=w123) -> (x+y=w124:dbl)
            n35 = Build Array(w120, w121) -> (w128:dbl[])
            n36 = Build Array(w118, w119) -> (w127:dbl[])
            n37 = property on="Stage Position" class="XYGraph (strict)"("XScale.Maximum"=w125, "XScale.Minimum"=w126, "YScale.Maximum"=w124, "YScale.Minimum"=w122, "XScale.MarkerVals[]"=w128, "YScale.MarkerVals[]"=w127) -> ()  [unwired: 2 in, 2 out]
          }
          event "Move to Start": Value Change {
            n38 = event-data() -> ()  [unwired: 1 in, 6 out]
          }
          event "Left": Value Change {
            w131 = 0.0  # Y Start
            w133 = sgl 0.0  # X Start
            w136 = 1.0  # Offset
            n39 = event-data() -> ()  [unwired: 1 in, 6 out]
            n40 = local read "X Max Stage"() -> (w134:dbl)
            n41 = local read "Y Maximum"() -> (w132:dbl)
            n42 = Add(x=w136, y=w134) -> (x+y=w138:dbl)
            n43 = Subtract(x=w133, y=w136) -> (x-y=w139:dbl)
            n44 = Subtract(x=w131, y=w136) -> (x-y=w135:dbl)
            n45 = Add(x=w132, y=w136) -> (x+y=w137:dbl)
            n46 = Build Array(w133, w134) -> (w141:dbl[])
            n47 = Build Array(w131, w132) -> (w140:dbl[])
            n48 = property on="Stage Position" class="XYGraph (strict)"("XScale.Maximum"=w138, "XScale.Minimum"=w139, "YScale.Maximum"=w137, "YScale.Minimum"=w135, "XScale.MarkerVals[]"=w141, "YScale.MarkerVals[]"=w140) -> ()  [unwired: 2 in, 2 out]
          }
          event "Right": Value Change {
            w143 = 0.0  # Y Start
            w145 = sgl 0.0  # X Start
            w148 = 1.0  # Offset
            n49 = event-data() -> ()  [unwired: 1 in, 6 out]
            n50 = local read "X Max Stage"() -> (w146:dbl)
            n51 = local read "Y Maximum"() -> (w144:dbl)
            n52 = Add(x=w148, y=w146) -> (x+y=w150:dbl)
            n53 = Subtract(x=w145, y=w148) -> (x-y=w151:dbl)
            n54 = Subtract(x=w143, y=w148) -> (x-y=w147:dbl)
            n55 = Add(x=w144, y=w148) -> (x+y=w149:dbl)
            n56 = Build Array(w145, w146) -> (w153:dbl[])
            n57 = Build Array(w143, w144) -> (w152:dbl[])
            n58 = property on="Stage Position" class="XYGraph (strict)"("XScale.Maximum"=w150, "XScale.Minimum"=w151, "YScale.Maximum"=w149, "YScale.Minimum"=w147, "XScale.MarkerVals[]"=w153, "YScale.MarkerVals[]"=w152) -> ()  [unwired: 2 in, 2 out]
          }
          event "Zero": Value Change {
            w155 = 0.0  # Y Start
            w157 = sgl 0.0  # X Start
            w160 = 1.0  # Offset
            n59 = event-data() -> ()  [unwired: 1 in, 6 out]
            n60 = local read "X Max Stage"() -> (w158:dbl)
            n61 = local read "Y Maximum"() -> (w156:dbl)
            n62 = Add(x=w160, y=w158) -> (x+y=w162:dbl)
            n63 = Subtract(x=w157, y=w160) -> (x-y=w163:dbl)
            n64 = Subtract(x=w155, y=w160) -> (x-y=w159:dbl)
            n65 = Add(x=w156, y=w160) -> (x+y=w161:dbl)
            n66 = Build Array(w157, w158) -> (w165:dbl[])
            n67 = Build Array(w155, w156) -> (w164:dbl[])
            n68 = property on="Stage Position" class="XYGraph (strict)"("XScale.Maximum"=w162, "XScale.Minimum"=w163, "YScale.Maximum"=w161, "YScale.Minimum"=w159, "XScale.MarkerVals[]"=w165, "YScale.MarkerVals[]"=w164) -> ()  [unwired: 2 in, 2 out]
          }
          event "Stop Motion": Value Change {
            n69 = event-data() -> ()  [unwired: 1 in, 6 out]
          }
          event "Start Stage": Value Change {
            n70 = event-data() -> ()  [unwired: 1 in, 6 out]
            n71 = local write "Machine Mode"(T5."Scanning Mode" ("Machine Mode")) -> ()
          }
          event "X Start", "X End", "Y Start", "Y End", "Y Step Size", "X Step Size", "Scan Mode": Value Change {
            n72 = event-data() -> ()  [unwired: 1 in, 6 out]
            n73 = local write "Machine Mode"(T5."Normal" ("Machine Mode")) -> ()
          }
          event "Speed Control (mm/s)": Value Change {
            n74 = event-data() -> ()  [unwired: 1 in, 6 out]
          }
          event "Outline": Value Change {
            n75 = event-data() -> ()  [unwired: 1 in, 6 out]
            n76 = case shown="True" "Outline" {
              tunnel: [StageOptions."Idle" StageOptions."GenerateMotionPoints"] -> w174
              frame False {
              }
              frame True {
                n77 = local write "Machine Mode"(T5."Perimeter Mode" ("Machine Mode")) -> ()
              }
            }
          }
          event "AbsMove": Value Change {
            w178 = 0.0  # Y Start
            w180 = sgl 0.0  # X Start
            w183 = 1.0  # Offset
            n78 = event-data() -> ()  [unwired: 1 in, 6 out]
            n79 = local read "X Max Stage"() -> (w181:dbl)
            n80 = local read "Y Maximum"() -> (w179:dbl)
            n81 = Add(x=w183, y=w181) -> (x+y=w185:dbl)
            n82 = Subtract(x=w180, y=w183) -> (x-y=w186:dbl)
            n83 = Subtract(x=w178, y=w183) -> (x-y=w182:dbl)
            n84 = Add(x=w179, y=w183) -> (x+y=w184:dbl)
            n85 = Build Array(w180, w181) -> (w188:dbl[])
            n86 = Build Array(w178, w179) -> (w187:dbl[])
            n87 = property on="Stage Position" class="XYGraph (strict)"("XScale.Maximum"=w185, "XScale.Minimum"=w186, "YScale.Maximum"=w184, "YScale.Minimum"=w182, "XScale.MarkerVals[]"=w188, "YScale.MarkerVals[]"=w187) -> ()  [unwired: 2 in, 2 out]
          }
        }
        n88 = case shown="True" w96 {
          frame False {
          }
          frame True {
            # "Trigger the Time Output\nFor the default values"
            n89 = property on="Scan Mode" class="Enum (strict)"() -> ("Value"=w101:enum16{"Raster", "Serpentine"})  [unwired: 2 in, 2 out]
            n90 = property on="Scan Mode" class="Enum (strict)"("Val(Sgnl)"=w101) -> ()  [unwired: 2 in, 2 out]
            n91 = local write "Machine Mode"(T5."Normal" ("Machine Mode")) -> ()
          }
        }
      }
      frame "Init" {
        w202 = 100  # numSteps = 1mm
        w203 = TRUE  # Correction File Path Option
        n92 = call "CloseDevices.vi"("error in (no error)"=w193, "Close"=TRUE, "Ids"=i32[] [1, 2]) -> ("error out"=w192:errorcluster)  [unwired: 8 in]
        n93 = case shown="False" w203 {
          tunnel: ["Correction Table Path (Hidden)" w209] -> w204
          frame False {
          }
          frame True {
            w210 = path "Corr_table_8MT173-25.tbl"  # File Name
            n94 = Current VI's Path() -> (path=w212:path)
            n95 = Build Path(base path=w212, name or relative path=path "") -> (appended path=w211:path)
            n96 = Build Path(base path=w211, name or relative path=w210) -> (appended path=w209:path)
          }
        }
        n97 = call "Find Controllers.vi"("error in (no error)"=w192) -> ("error out"=w206:errorcluster, "Names"=w207:string[])  [unwired: 8 in, 1 out]
        n98 = call "OpenDevices.vi"("error In"=w206, "Names"=w207) -> ("error out"=w205:errorcluster, "Serial nos"=→"Serial nos":u32[], "IDs"=w200:i32[])  [unwired: 6 in]
        "IDs" <- w200
        n99 = call "CalibrateStage.vi"("error in (no error)"=w205, "numSteps = 1mm"=w202, "Correction Table Path"=w204, "IDs"=w200) -> ("error out"=w195:errorcluster, "Calibration"=→"Calibration":cluster{dbl, "MicrostepMode":u32}[])  [unwired: 2 in, 4 out]
        n100 = Unbundle By Name(w195) -> ("status"=w197:bool)
        n101 = Not(x=w197) -> (.not. x?=w196:bool)
      }
      frame "Set Speed" {
        n102 = local read "IDs"() -> (w217:i32[])
        n103 = local read "Calibration"() -> (w216:cluster{dbl, "MicrostepMode":u32}[])
        n104 = call "SetMoveSettings.vi"("Mode"=SettingCtrlOptions."Set X and Y", "error in (no error)"=w219, "Calibration"=w216, "Speed"="Speed Control (mm/s)", "IDs"=w217) -> ("error out"=w218:errorcluster)  [unwired: 4 in, 2 out]
      }
      frame "GenerateMotionPoints" {
        n105 = local read "Calibration"() -> (w247:cluster{dbl, "MicrostepMode":u32}[])
        n106 = Subtract(x="X End", y="X Start") -> (x-y=w236:sgl)
        n107 = Divide(x=w236, y="X Step Size") -> (x/y=w252:sgl)
        n108 = Subtract(x="Y End", y="Y Start") -> (x-y=w234:sgl)
        n109 = Increment(x=w252) -> (x+1=w239:sgl)
        n110 = Divide(x=w234, y="Y Step Size") -> (x/y=w249:sgl)
        n111 = To Long Integer(number=w239) -> (32bit integer=w251:i32)
        n112 = Increment(x=w249) -> (x+1=w238:sgl)
        n113 = To Long Integer(number=w238) -> (32bit integer=w248:i32)
        n114 = call "GenerateScanEndPts.vi"("X Start"="X Start", "Mode"="Scan Mode", "Calibration In"=w247, "X End"="X End", "Y Start"="Y Start", "Y End"="Y End", "error in"=w256, "Line Count"=w248, "Pixel Count"=w251, "EdgePt/nPixelMap"="EdgePt/nPixelMap") -> ("Coordinate Array"=→"Coordinate Array":sgl[][], "X Pixel Count"=w230:u64, "Step Sizes"=w232:sgl[], "Y Pixel Count"=w229:u64, "error out"=w257:errorcluster)  [unwired: 1 in]
        "Line Count" <- w229
        "Pixel Count" <- w230
        "Step Sizes" <- w232
        n115 = call "PeripheralCoordinates.vi"("Y End"="Y End", "Y Start"="Y Start", "X End"="X End", "X Start"="X Start") -> ("Coordinate Array"=→"Peripheral Coordis":sgl[][])  [unwired: 7 in]
        n116 = local read "Speed Control (mm/s)"() -> (w233:sgl)
        n117 = Multiply(x=w229, y=w230) -> (x*y=w226:u64)
        "Total Pixels" <- w226
        n118 = Index Array(array=w232) -> (element #1=→"X Step Size (R)":sgl, element #2=→"Y Step Size (R)":sgl)  [unwired: 2 in]
        n119 = call "Calculate Scan Time.vi"("Step Sizes"=w232, "Scan Mode"="Scan Mode", "Speed Control (mm/s)"=w233, "Line Count"=w229, "Pixel Count"=w230) -> ("TimeString"=→"Scan Time (Approx.)":string, "total time (sec)"=→"total time (sec)":sgl)  [unwired: 2 in, 3 out]
        n120 = case shown="\"Scanning Mode\"" "Machine Mode" {
          tunnel: [StageOptions."Scan_Start" StageOptions."Scan_Start" StageOptions."Idle"] -> w241
          frame "Scanning Mode" {
          }
          frame "Perimeter Mode" {
          }
          frame "Normal", Default {
          }
        }
        n121 = Initialize Array(0.0 ("element"), w226) -> (w224:dbl[])
        "AmplitudeArray" <- w224
        "IndexArray" <- w224
        n122 = call <extravilib>:"Write.vi"("element"=w224) -> ("channel"=w223:T23)  [unwired: 1 out]
      }
      frame "Scan_Start" {
        n123 = call <vilib>:"Set Busy.vi"("error in (no error)"=w264) -> ("error out"=w263:errorcluster)  [unwired: 9 in, 1 out]
        n124 = stacked-sequence {
          seq-local: [_ w273 _ _ _ _ _] -> [_ _ _ _ _ _ w345]
          seq-local: [w267 _ _ _ _ _ _] -> [_ _ _ _ _ _ w346]
          seq-local: [_ _ _ _ w327 _ _] -> [_ _ _ _ _ _ w343]
          seq-local: [_ _ _ w299 _ _ _] -> [_ _ _ _ _ _ w344]
          seq-local: [_ _ _ _ _ w335 _] -> [_ _ _ _ _ _ w342]
          tunnel: w263 -> [_ _ _ _ _ _ w365]
          tunnel: [_ _ _ _ _ _ w359] -> w266
          tunnel: [_ _ _ _ _ _ w348] -> w265
          frame #0 {
            # "Start Generator"
            n125 = control-ref of="stop Gen"() -> (w269:refnum<vi>)
            n126 = control-ref of="Generator On"() -> (w271:refnum<vi>)
            n127 = control-ref of="Start Gen"() -> (w270:refnum<vi>)
            n128 = call "SwitchTillOn.vi"("Stop if On?"=TRUE, "Turn Off Button"=w269, "timeout"=u32 300000, "Turn On Button"=w270, "Turn On Indicator"=w271) -> ("Success?"=w267:bool)  [unwired: 6 in]
          }
          frame #1 {
            # "Start Digitizer"
            n129 = flat-sequence {
              tunnel: [w275] -> w274
              tunnel: w274 -> [w281]
              tunnel: [w281] -> w273
              frame #0 {
                n130 = control-ref of="Digitizer On"() -> (w278:refnum<vi>)
                n131 = control-ref of="Start Digi"() -> (w277:refnum<vi>)
                n132 = call "SwitchTillOn.vi"("Stop if On?"=FALSE, "timeout"=u32 5000, "Turn On Button"=w277, "Turn On Indicator"=w278) -> ("Success?"=w275:bool)  [unwired: 7 in]
              }
              frame #1 {
                n133 = local write "Digi Machine Mode"(DigiMachineStates."Scanning Mode" ("Digi Machine Mode")) -> ()
              }
              frame #2 {
                n134 = while {
                  stop <- w283 stop-if-true
                  n135 = local read "Digi Machine Mode"() -> (w284:T8)
                  n136 = Equal?(x=w284, y=DigiMachineStates."Scanning Mode") -> (x = y?=w283:bool)
                }
              }
            }
          }
          frame #2 {
            # "Reset Data Storing"
            n137 = while {
              stop <- w286 stop-if-true
              n138 = local read "FileStore State"() -> (w291:T11)
              n139 = local read "FileStore State"() -> (w289:T11)
              n140 = Equal?(x=w289, y=Data_Save_State."Close File" ("FileStore State")) -> (x = y?=w287:bool)
              n141 = Equal?(x=w291, y=Data_Save_State."Idle" ("FileStore State")) -> (x = y?=w290:bool)
              n142 = Or(x=w290, y=w287) -> (x .or. y?=w286:bool)
              n143 = Not(x=w286) -> (.not. x?=w285:bool)
              n144 = local write "Done Recording"(w285) -> ()
            }
          }
          frame #3 {
            w295 = T10 {"Wave Count"=0, "Wave"=[]} ("input cluster")
            # "Flush All Queue"
            n145 = Obtain Queue(name (unnamed)="AquiredDataFIFO_Wave", element data type=w295, create if not found? (T)=TRUE) -> (queue out=w296:refnum<queue>, error out=w297:errorcluster)  [unwired: 2 in, 1 out]
            n146 = Obtain Queue(name (unnamed)="AquiredDataFIFOCopy", element data type=w295, create if not found? (T)=TRUE, error in (no error)=w297) -> (queue out=w304:refnum<queue>, error out=w302:errorcluster)  [unwired: 1 in, 1 out]
            n147 = Obtain Queue(name (unnamed)="AquiredDataFIFO", element data type=T16 {"Wave Count"=0, "Amplitude"=0, "Index"=0} ("cluster"), create if not found? (T)=TRUE, error in (no error)=w302) -> (queue out=w305:refnum<queue>, error out=w303:errorcluster)  [unwired: 1 in, 1 out]
            n148 = while {
              tunnel: w305 -> [w326]
              tunnel: w304 -> [w325]
              shift-right: [w313] -> w301
              shift-left: w303 -> [w322]
              tunnel: w296 -> [w310]
              stop <- w315 stop-if-true
              n149 = Flush Queue(queue=w326, error in (no error)=w322) -> (queue out=w321:refnum<queue>, error out=w323:errorcluster)  [unwired: 1 out]
              n150 = Get Queue Status(queue=w321) -> (# elements in queue=w317:i32)  [unwired: 2 in, 7 out]
              n151 = Flush Queue(queue=w325, error in (no error)=w323) -> (queue out=w319:refnum<queue>, error out=w324:errorcluster)  [unwired: 1 out]
              n152 = Get Queue Status(queue=w319, error in (no error)=w324) -> (error out=w320:errorcluster, # elements in queue=w318:i32)  [unwired: 1 in, 6 out]
              n153 = Flush Queue(queue=w310, error in (no error)=w320) -> (queue out=w312:refnum<queue>, error out=w314:errorcluster)  [unwired: 1 out]
              n154 = Get Queue Status(queue=w312, error in (no error)=w314) -> (error out=w313:errorcluster, # elements in queue=w311:i32)  [unwired: 1 in, 6 out]
              n155 = Compound Arithmetic op=ADD(w311, w318, w317) -> (w316:i32)
              n156 = Equal To 0?(x=w316) -> (x = 0?=w315:bool)
            }
            n157 = Unbundle By Name(w301) -> ("status"=w300:bool)
            n158 = Not(x=w300) -> (.not. x?=w299:bool)
          }
          frame #4 {
            # "Open File"
            n159 = case shown="True" "Save to File" {
              tunnel: [TRUE ("Success?") w330] -> w327
              frame False {
              }
              frame True {
                n160 = while {
                  tunnel: [w331] -> w330
                  stop <- w331 stop-if-true
                  n161 = local read "FileStore State"() -> (w334:T11)
                  n162 = Equal?(x=w334, y=Data_Save_State."Append Data" ("FileStore State")) -> (x = y?=w331:bool)
                  n163 = Not(x=w331) -> (.not. x?=w332:bool)
                  n164 = local write "Record Data"(w331) -> ()
                  n165 = local write "Open File"(w332) -> ()
                }
              }
            }
          }
          frame #5 {
            # "Reset Wave Number Count"
            n166 = control-ref of="CountReset"() -> (w336:refnum<vi>)
            n167 = control-ref of="Wave Count Zero"() -> (w337:refnum<vi>)
            n168 = call "SwitchTillOn.vi"("Stop if On?"=FALSE, "timeout"=u32 5000, "Turn On Button"=w336, "Turn On Indicator"=w337) -> ("Success?"=w335:bool)  [unwired: 7 in]
          }
          frame #6 {
            w362 = 0.0 ("element")
            w371 = 1.0  # Offset
            # "Draw Markers To Indicate the Scan Area"
            n169 = property on="X End" class="DigNum (strict)"() -> ("Value"=w370:sgl)  [unwired: 2 in, 2 out]
            n170 = property on="X Start" class="DigNum (strict)"() -> ("Value"=w369:sgl)  [unwired: 2 in, 2 out]
            n171 = property on="Y End" class="DigNum (strict)"() -> ("Value"=w366:sgl)  [unwired: 2 in, 2 out]
            n172 = property on="Y Start" class="DigNum (strict)"() -> ("Value"=w368:sgl)  [unwired: 2 in, 2 out]
            n173 = Add(x=w371, y=w370) -> (x+y=w373:dbl)
            n174 = Subtract(x=w369, y=w371) -> (x-y=w374:dbl)
            n175 = Add(x=w366, y=w371) -> (x+y=w372:dbl)
            n176 = Subtract(x=w368, y=w371) -> (x-y=w367:dbl)
            n177 = Build Array(w369, w370) -> (w376:sgl[])
            n178 = Build Array(w368, w366) -> (w375:sgl[])
            n179 = property on="Stage Position" class="XYGraph (strict)"(error in=w365, "XScale.Maximum"=w373, "XScale.Minimum"=w374, "YScale.Maximum"=w372, "YScale.Minimum"=w367, "XScale.MarkerVals[]"=w376, "YScale.MarkerVals[]"=w375) -> (error out=w351:errorcluster)  [unwired: 1 in, 1 out]
            n180 = local read "EdgePt/nPixelMap"() -> (w355:bool)
            n181 = local read "IDs"() -> (w358:i32[])
            n182 = local read "Step Sizes"() -> (w356:sgl[])
            n183 = local read "Calibration"() -> (w357:cluster{dbl, "MicrostepMode":u32}[])
            n184 = call "SetSyncSettings.vi"("Periodic/nPointScan"=w355, "X SyncOut Enabled"=FALSE, "Y SyncOut Enabled"=FALSE, "error in (no error)"=w351, "Calibration"=w357, "Step Sizes(mm)"=w356, "IDs"=w358) -> ("error out"=w352:errorcluster)  [unwired: 3 in, 1 out]
            n185 = local read "IDs"() -> (w360:i32[])
            n186 = local read "Calibration"() -> (w361:cluster{dbl, "MicrostepMode":u32}[])
            n187 = local write "Next Coordinate Index"(0 ("Next Coordinate Index")) -> ()
            n188 = Build Array(w362, w362) -> (w363:dbl[])
            n189 = Compound Arithmetic op=AND(w346, w345, w344, w343, w342) -> (w341:bool)
            n190 = call "PositionControlRelative.vi"("Mode"=PosCtrlOptions."Both X and Y", "error in (no error)"=w352, "Calibration"=w361, "Move to"=w363, "IDs"=w360) -> ("error out"=w359:errorcluster)  [unwired: 4 in, 2 out]
            n191 = Not(x=w341) -> (.not. x?=w340:bool)
            n192 = Select(t=StageOptions."Scan_Get Pos", s=w341, f=StageOptions."Idle") -> (s? t:f=w348:T6)
            n193 = local write "Imaging"(w341) -> ()
            n194 = call "Display Message to User5"("Enable"=w340) -> ()  [unwired: 9 in, 2 out]
          }
        }
        n195 = call <vilib>:"Unset Busy.vi"("error in (no error)"=w266) -> ("error out"=w262:errorcluster)  [unwired: 10 in]
      }
      frame "Scan_Get Pos" {
        n196 = local read "IDs"() -> (w390:i32[])
        n197 = local read "Calibration"() -> (w391:cluster{dbl, "MicrostepMode":u32}[])
        n198 = call "PositionControl.vi"("Mode"=PosCtrlOptions."Read Pos", "error in (no error)"=w393, "Calibration"=w391, "IDs"=w390) -> ("error out"=w392:errorcluster, "Moving?"=w382:bool, "Position"=w385:sgl[])  [unwired: 4 in, 1 out]
        n199 = local write "Moving?"(w382) -> ()
        n200 = Index Array(array=w385, index #1=0 ("index"), index #2=1 ("index")) -> (element #1=w379:sgl, element #2=w378:sgl)
        n201 = local write "X Position"(w379) -> ()
        n202 = local write "Y Position"(w378) -> ()
        n203 = Build Array(w379) -> (w388:sgl[])
        n204 = Build Array(w378) -> (w389:sgl[])
        n205 = Bundle(w388, w389) -> (w384:cluster{sgl[], sgl[]})  [unwired: 1 in]
        n206 = local write "Stage Position"(w384) -> ()
        n207 = property on="Stage Position" class="XYGraph (strict)"("Cursor.Cursor X"=w379, "Cursor.Cursor Y"=w378) -> ()  [unwired: 2 in, 2 out]
        n208 = Select(t=StageOptions."Scan_Get Pos", s=w382, f=StageOptions."Scan_SyncSet") -> (s? t:f=w383:T6)
      }
      frame "Scan_SyncSet" {
        n209 = local read "EdgePt/nPixelMap"() -> (w397:bool)
        n210 = local read "IDs"() -> (w405:i32[])
        n211 = local read "Step Sizes"() -> (w403:sgl[])
        n212 = local read "Calibration"() -> (w404:cluster{dbl, "MicrostepMode":u32}[])
        n213 = Quotient & Remainder(x="Next Coordinate Index", y=2) -> (x-y*floor(x/y)=w400:i32)  [unwired: 1 out]
        n214 = Not Equal To 0?(x=w400) -> (x != 0?=w398:bool)
        n215 = Compound Arithmetic op=OR(invert w397, w398) -> (w399:bool)
        n216 = call "SetSyncSettings.vi"("Periodic/nPointScan"=w397, "X SyncOut Enabled"=w399, "Y SyncOut Enabled"=FALSE, "error in (no error)"=w408, "Calibration"=w404, "Step Sizes(mm)"=w403, "IDs"=w405) -> ("error out"=w407:errorcluster)  [unwired: 3 in, 1 out]
      }
      frame "Scan_MoveNext" {
        n217 = flat-sequence {
          tunnel: w422 -> [w425]
          tunnel: [w425] -> w414
          tunnel: [w424] -> w413
          tunnel: [w423] -> w411
          tunnel: [w433] -> w420
          tunnel: [w430] -> w419
          tunnel: [w429] -> w415
          tunnel: w414 -> [w434]
          tunnel: w413 -> [w429]
          tunnel: [w428] -> w412
          tunnel: w411 -> [w428]
          tunnel: [w444] -> w410
          tunnel: [w445] -> w421
          tunnel: w412 -> [w437]
          tunnel: w415 -> [w441]
          tunnel: w419 -> [w442]
          tunnel: w420 -> [w445]
          frame #0 {
            n218 = local read "Machine Mode"() -> (w423:T5)
            n219 = case shown="\"Perimeter Mode\"" w423 {
              tunnel: [w426 w427] -> w424
              frame "Scanning Mode", Default {
                n220 = local read "Coordinate Array"() -> (w426:sgl[][])
              }
              frame "Perimeter Mode" {
                n221 = local read "Peripheral Coordis"() -> (w427:sgl[][])
              }
            }
          }
          frame #1 {
            n222 = local read "IDs"() -> (w432:i32[])
            n223 = local read "Calibration"() -> (w431:cluster{dbl, "MicrostepMode":u32}[])
            n224 = local read "Next Coordinate Index"() -> (w430:i32)
            n225 = Index Array(array=w429, index (row)=w430) -> (element=w435:sgl[])  [unwired: 1 in]
            n226 = call "PositionControl.vi"("Mode"=PosCtrlOptions."Both X and Y", "error in (no error)"=w434, "Calibration"=w431, "Move to"=w435, "IDs"=w432) -> ("error out"=w433:errorcluster)  [unwired: 3 in, 3 out]
          }
          frame #2 {
            n227 = Increment(x=w442) -> (x+1=w438:i32)
            n228 = Matrix Size(0:w441) -> (1:w440:i32)  [unwired: 1 out]
            n229 = Greater?(x=w438, y=w440) -> (0:w439:bool)
            n230 = case shown="True" w439 {
              selector: w439 -> [w446 _]
              tunnel: w438 -> [w447 w450]
              tunnel: [w447 w449] -> w443
              tunnel: [w446 w448] -> w444
              tunnel: w437 -> [_ w451]
              frame False {
              }
              frame True {
                n231 = case shown="\"Perimeter Mode\"" w451 {
                  tunnel: w450 -> [w453 _]
                  tunnel: [w453 0] -> w449
                  tunnel: [TRUE ("x > y?") w455] -> w448
                  frame "Scanning Mode", Default {
                  }
                  frame "Perimeter Mode" {
                    n232 = local read "Outline"() -> (w456:bool)
                    n233 = Not(x=w456) -> (.not. x?=w455:bool)
                  }
                }
              }
            }
            n234 = local write "Next Coordinate Index"(w443) -> ()
          }
        }
        n235 = Not(x=w410) -> (.not. x?=w409:bool)
        n236 = Select(t=StageOptions."Scan_Complete", s=w410, f=StageOptions."Scan_Get Pos") -> (s? t:f=w418:T6)
      }
      frame "Scan_Complete" {
        n237 = stacked-sequence {
          tunnel: [w474 _] -> w461
          tunnel: w459 -> [w466 _]
          frame #0 {
            w463 = FALSE ("Y SyncOut Enabled")
            w472 = 0.0 ("element")
            # "Trigger After Reaching Zero to compensate For a Missed Trigger (If There)"
            n238 = local read "IDs"() -> (w469:i32[])
            n239 = local read "Step Sizes"() -> (w467:sgl[])
            n240 = local read "Calibration"() -> (w468:cluster{dbl, "MicrostepMode":u32}[])
            n241 = call "SetSyncSettings.vi"("Periodic/nPointScan"=w463, "X SyncOut Enabled"=TRUE, "Y SyncOut Enabled"=w463, "error in (no error)"=w466, "Calibration"=w468, "Step Sizes(mm)"=w467, "IDs"=w469) -> ("error out"=w465:errorcluster)  [unwired: 3 in, 1 out]
            n242 = local write "Machine Mode"(T5."Normal" ("Machine Mode")) -> ()
            n243 = local read "IDs"() -> (w470:i32[])
            n244 = local read "Calibration"() -> (w471:cluster{dbl, "MicrostepMode":u32}[])
            n245 = Build Array(w472, w472) -> (w473:dbl[])
            n246 = call "PositionControl.vi"("Mode"=PosCtrlOptions."Both X and Y", "error in (no error)"=w465, "Calibration"=w471, "Move to"=w473, "IDs"=w470) -> ("error out"=w474:errorcluster)  [unwired: 3 in, 3 out]
          }
          frame #1 {
            n247 = local write "Digi Machine Mode"(DigiMachineStates."Idle Mode" ("Digi Machine Mode")) -> ()
          }
        }
      }
      frame "Cmd_MoveAbs" {
        n248 = local read "IDs"() -> (w482:i32[])
        n249 = local read "Calibration"() -> (w481:cluster{dbl, "MicrostepMode":u32}[])
        n250 = Build Array("X Position Abs", "Y Position Abs") -> (w480:dbl[])
        n251 = call "PositionControl.vi"("Mode"=PosCtrlOptions."Both X and Y", "error in (no error)"=w484, "Calibration"=w481, "Move to"=w480, "IDs"=w482) -> ("error out"=w483:errorcluster)  [unwired: 3 in, 3 out]
      }
      frame "Cmd_MoveStart" {
        n252 = local read "X Start"() -> (w487:sgl)
        n253 = local read "Y Start"() -> (w486:sgl)
        n254 = local read "IDs"() -> (w491:i32[])
        n255 = local read "Calibration"() -> (w490:cluster{dbl, "MicrostepMode":u32}[])
        n256 = Build Array(w487, w486) -> (w489:sgl[])
        n257 = call "PositionControl.vi"("Mode"=PosCtrlOptions."Both X and Y", "error in (no error)"=w493, "Calibration"=w490, "Move to"=w489, "IDs"=w491) -> ("error out"=w492:errorcluster)  [unwired: 3 in, 3 out]
      }
      frame "Cmd_CloseControllers" {
        n258 = local read "IDs"() -> (w496:i32[])
        n259 = for {
          shift-right: [w503] -> w500
          shift-left: w498 -> [w502]
          tunnel: w496 -> [w501] mode=indexing
          n260 = call "command stop.vi"("error in (no error)"=w502, "id"=w501) -> ("error out"=w503:errorcluster)  [unwired: 8 in, 1 out]
        }
        n261 = call "CloseDevices.vi"("error in (no error)"=w500, "Close"=TRUE, "Ids"=w496) -> ("error out"=w499:errorcluster)  [unwired: 8 in]
      }
      frame "Cmd_MoveUp" {
        n262 = local read "Move Step"() -> (w507:dbl)
        n263 = local read "IDs"() -> (w506:i32[])
        n264 = local read "Calibration"() -> (w505:cluster{dbl, "MicrostepMode":u32}[])
        n265 = Build Array(0.0 ("element"), w507) -> (w509:dbl[])
        n266 = call "PositionControlRelative.vi"("Mode"=PosCtrlOptions."Move Y", "error in (no error)"=w511, "Calibration"=w505, "Move to"=w509, "IDs"=w506) -> ("error out"=w510:errorcluster)  [unwired: 4 in, 2 out]
      }
      frame "Cmd_MoveDown" {
        n267 = local read "Move Step"() -> (w517:dbl)
        n268 = local read "IDs"() -> (w515:i32[])
        n269 = local read "Calibration"() -> (w514:cluster{dbl, "MicrostepMode":u32}[])
        n270 = Negate(x=w517) -> (-x=w516:dbl)
        n271 = Build Array(0.0 ("element"), w516) -> (w519:dbl[])
        n272 = call "PositionControlRelative.vi"("Mode"=PosCtrlOptions."Move Y", "error in (no error)"=w521, "Calibration"=w514, "Move to"=w519, "IDs"=w515) -> ("error out"=w520:errorcluster)  [unwired: 4 in, 2 out]
      }
      frame "Cmd_MoveLeft" {
        n273 = local read "Move Step"() -> (w528:dbl)
        n274 = local read "IDs"() -> (w524:i32[])
        n275 = local read "Calibration"() -> (w525:cluster{dbl, "MicrostepMode":u32}[])
        n276 = Negate(x=w528) -> (-x=w527:dbl)
        n277 = Build Array(w527, 0.0 ("element")) -> (w529:dbl[])
        n278 = call "PositionControlRelative.vi"("Mode"=PosCtrlOptions."Move X", "error in (no error)"=w531, "Calibration"=w525, "Move to"=w529, "IDs"=w524) -> ("error out"=w530:errorcluster)  [unwired: 4 in, 2 out]
      }
      frame "Cmd_MoveRight" {
        n279 = local read "Move Step"() -> (w537:dbl)
        n280 = local read "IDs"() -> (w535:i32[])
        n281 = local read "Calibration"() -> (w534:cluster{dbl, "MicrostepMode":u32}[])
        n282 = Build Array(w537, 0.0 ("element")) -> (w538:dbl[])
        n283 = call "PositionControlRelative.vi"("Mode"=PosCtrlOptions."Move X", "error in (no error)"=w540, "Calibration"=w534, "Move to"=w538, "IDs"=w535) -> ("error out"=w539:errorcluster)  [unwired: 4 in, 2 out]
      }
      frame "Cmd_MoveZero" {
        w545 = 0.0 ("element")
        n284 = local read "IDs"() -> (w543:i32[])
        n285 = local read "Calibration"() -> (w544:cluster{dbl, "MicrostepMode":u32}[])
        n286 = Build Array(w545, w545) -> (w546:dbl[])
        n287 = call "PositionControl.vi"("Mode"=PosCtrlOptions."Both X and Y", "error in (no error)"=w548, "Calibration"=w544, "Move to"=w546, "IDs"=w543) -> ("error out"=w547:errorcluster)  [unwired: 3 in, 3 out]
      }
      frame "Cmd_GetPos" {
        n288 = local read "IDs"() -> (w560:i32[])
        n289 = local read "Calibration"() -> (w561:cluster{dbl, "MicrostepMode":u32}[])
        n290 = call "PositionControl.vi"("Mode"=PosCtrlOptions."Read Pos", "error in (no error)"=w563, "Calibration"=w561, "IDs"=w560) -> ("error out"=w562:errorcluster, "Moving?"=→"Moving?":bool, "Position"=w554:sgl[])  [unwired: 4 in, 1 out]
        n291 = Index Array(array=w554, index #1=0 ("index"), index #2=1 ("index")) -> (element #1=w551:sgl, element #2=w550:sgl)
        n292 = local write "X Position"(w551) -> ()
        n293 = local write "Y Position"(w550) -> ()
        n294 = Build Array(w551) -> (w558:sgl[])
        n295 = Build Array(w550) -> (w559:sgl[])
        n296 = Bundle(w558, w559) -> (→"Stage Position":cluster{sgl[], sgl[]})  [unwired: 1 in]
        n297 = property on="Stage Position" class="XYGraph (strict)"("Cursor.Cursor X"=w551, "Cursor.Cursor Y"=w550) -> ()  [unwired: 2 in, 2 out]
      }
      frame "Cmd_Stop" {
        n298 = local read "IDs"() -> (w566:i32[])
        n299 = for {
          shift-right: [w571] -> w568
          shift-left: w567 -> [w570]
          tunnel: w566 -> [w569] mode=indexing
          n300 = call "command stop.vi"("error in (no error)"=w570, "id"=w569) -> ("error out"=w571:errorcluster)  [unwired: 8 in, 1 out]
        }
      }
      frame "Sync_On" {
        n301 = local read "EdgePt/nPixelMap"() -> (w574:bool)
        n302 = local read "IDs"() -> (w577:i32[])
        n303 = local read "Step Sizes"() -> (w575:sgl[])
        n304 = local read "Calibration"() -> (w576:cluster{dbl, "MicrostepMode":u32}[])
        n305 = call "SetSyncSettings.vi"("Periodic/nPointScan"=w574, "X SyncOut Enabled"=TRUE, "Y SyncOut Enabled"=FALSE, "error in (no error)"=w580, "Calibration"=w576, "Step Sizes(mm)"=w575, "IDs"=w577) -> ("error out"=w579:errorcluster)  [unwired: 3 in, 1 out]
      }
      frame "Sync_Off" {
        n306 = local read "EdgePt/nPixelMap"() -> (w583:bool)
        n307 = local read "IDs"() -> (w586:i32[])
        n308 = local read "Step Sizes"() -> (w584:sgl[])
        n309 = local read "Calibration"() -> (w585:cluster{dbl, "MicrostepMode":u32}[])
        n310 = call "SetSyncSettings.vi"("Periodic/nPointScan"=w583, "X SyncOut Enabled"=FALSE, "Y SyncOut Enabled"=FALSE, "error in (no error)"=w589, "Calibration"=w585, "Step Sizes(mm)"=w584, "IDs"=w586) -> ("error out"=w588:errorcluster)  [unwired: 3 in, 1 out]
      }
      frame "Stop Motion" {
        w592 = TRUE ("Close")
        n311 = local read "IDs"() -> (w594:i32[])
        n312 = for {
          shift-right: [w600] -> w597
          shift-left: w595 -> [w599]
          tunnel: w594 -> [w598] mode=indexing
          n313 = call "command stop.vi"("error in (no error)"=w599, "id"=w598) -> ("error out"=w600:errorcluster)  [unwired: 8 in, 1 out]
        }
        n314 = call "CloseDevices.vi"("error in (no error)"=w597, "Close"=w592, "Ids"=w594) -> ("error out"=w596:errorcluster)  [unwired: 8 in]
        n315 = local write "Moving?"(FALSE ("Moving?")) -> ()
        n316 = local write "Machine Mode"(T5."Normal" ("Machine Mode")) -> ()
      }
      frame "CloseApplication" {
        w602 = TRUE ("Close")
        n317 = local read "IDs"() -> (w605:i32[])
        n318 = local write "Moving?"(FALSE ("Moving?")) -> ()
        n319 = for {
          shift-right: [w611] -> w608
          shift-left: w606 -> [w610]
          tunnel: w605 -> [w609] mode=indexing
          n320 = call "command stop.vi"("error in (no error)"=w610, "id"=w609) -> ("error out"=w611:errorcluster)  [unwired: 8 in, 1 out]
        }
        n321 = call "CloseDevices.vi"("error in (no error)"=w608, "Close"=w602, "Ids"=w605) -> ("error out"=w607:errorcluster)  [unwired: 8 in]
        n322 = local write "Machine Mode"(T5."Normal" ("Machine Mode")) -> ()
      }
    }
    "Scan Running" <- w71
    n323 = local read "Serial nos"() -> (w77:u32[])
    n324 = call <instrlib>:"Synchronous Latch.vi"("clear"=w85, "set"=w87) -> ("out"=w86:bool)  [unwired: 9 in]
    n325 = call <instrlib>:"Synchronous Latch.vi"("clear"=w72, "set"=w74) -> ("out"=→"Scan Complete":bool)  [unwired: 9 in]
    n326 = Not(x=w86) -> (.not. x?=w79:bool)
    n327 = Greater Than 0?(x=w77) -> (x > 0?=w76:bool[])
    n328 = Or(x=w91, y="Stop Stage") -> (x .or. y?=w88:bool)
    n329 = And Array Elements(Boolean array=w76) -> (logical AND=w75:bool)
    n330 = Select(t=StageOptions."Stop Motion", s=w88, f=w89) -> (s? t:f=w82:T6)
    n331 = And(x=w75, y=w79) -> (x .and. y?=→"Controller Open?":bool)
    n332 = Select(t=StageOptions."CloseApplication", s="Stop Stage App", f=w82) -> (s? t:f=w83:T6)
    "Stage Status" <- w94
  }
  "Error Out Stage" <- w24
  n333 = timed-loop "Generator Control" {
    shift-right: [w620] -> _
    shift-left: Generator_States."Idle" -> [w623]
    shift-right: [w621] -> w38
    shift-left: errorcluster {"status"=FALSE, "code"=0, "source"=""} ("error in") -> [w622]
    timing: w58 -> [_]
    timing-out: [_] -> w57
    stop <- w612 stop-if-true
    n334 = node-c288() -> ()  [unwired: 1 in, 1 out]
    n335 = case shown="\"InitGen\"" w623 {
      tunnel: [w626 Generator_States."InitGen" Generator_States."Idle" Generator_States."Idle" Generator_States."Idle" Generator_States."Idle"] -> w619
      tunnel: w622 -> [w634 w647 w661 w667 w672 w677]
      tunnel: [w634 w641 w650 w666 w671 w676] -> w621
      tunnel: [_ _ w648 _ _ _] -> w617
      tunnel: [w633 _ _ _ TRUE ("x .or. y?") w673] -> w616
      tunnel: [_ _ _ _ _ w673] -> w612
      frame "Idle", Default {
        n336 = Build Array("Send vi Trig", "Start Gen", "stop Gen", FALSE ("element")) -> (w632:bool[])
        n337 = Boolean Array To Number(Boolean array=w632) -> (number=w627:u32)
        n338 = case shown="4" w627 {
          tunnel: [Generator_States."Idle" ("f") Generator_States."SendVITrig" Generator_States."GenerateWaveArray" Generator_States."CloseGen"] -> w626
          frame 0, Default {
          }
          frame 1 {
          }
          frame 2 {
          }
          frame 4 {
          }
        }
        n339 = First Call?() -> (First Call?: T/F=w633:bool)
      }
      frame "GenerateWaveArray" {
        n340 = call "WaveSynthV2.vi"("error in"=w647, "Default Wave"="Use Default Wave Settings") -> ("error out"=w641:errorcluster, "Waves per Pixel 2"=→"Waves per Pixel":u32, "Sampling Frequency (Hz) 2"=→"Sampling Frequency (Hz)":u64, "Amplitudes"=→"Amplitudes" →"Input Waveform":dbl[], "Offset Factor 2"=→"Offset Factor":dbl, "Gain"=→"Gain":dbl)  [unwired: 2 in]
      }
      frame "InitGen" {
        n341 = local read "Gain"() -> (w656:dbl)
        n342 = local read "Amplitudes"() -> (w657:dbl[])
        n343 = local read "Sampling Frequency (Hz)"() -> (w659:u64)
        n344 = local read "Waves per Pixel"() -> (w658:u32)
        n345 = local read "Offset Factor"() -> (w655:dbl)
        n346 = call "InitGen.vi"("Offset"=w655, "Gain"=w656, "Ext/nViTrig"="Ext/nViTrig", "Waveform Data Array"=w657, "error in (no error)"=w661, "Wave Per Pixel"=w658, "Sample Rate (Samp/s)"=w659, "FGEN Resource Name"="Generator  Port") -> ("error out"=w653:errorcluster, "Actual Sample Rate"=→"Actual Sample Rate":dbl, "reference out"=w652:refnum<k15>)  [unwired: 1 in]
        n347 = call "EnableOutput.vi"("error in (no error)"=w653, "FGEN Resource Name"=w652) -> ("error out"=w650:errorcluster)  [unwired: 8 in, 1 out]
        n348 = Unbundle By Name(w650) -> ("status"=w649:bool)
        n349 = Not(x=w649) -> (.not. x?=w648:bool)
      }
      frame "SendVITrig" {
        n350 = local read "Generator  Port"() -> (w664:refnum<k15>)
        n351 = call "SendTrig.vi"("error in (no error)"=w667, "Send vi Trig"=TRUE, "Instrument Handle"=w664) -> ("error out"=w666:errorcluster)  [unwired: 7 in, 1 out]
      }
      frame "CloseGen" {
        n352 = local read "Generator  Port"() -> (w670:refnum<k15>)
        n353 = call "CloseGen.vi"("error in (no error)"=w672, "Instrument Handle"=w670) -> ("error out"=w671:errorcluster)  [unwired: 9 in]
      }
      frame "CloseApp" {
        w673 = TRUE ("x .or. y?")
        n354 = local read "Generator  Port"() -> (w675:refnum<k15>)
        n355 = call "CloseGen.vi"("error in (no error)"=w677, "Instrument Handle"=w675) -> ("error out"=w676:errorcluster)  [unwired: 9 in]
      }
    }
    n356 = call <instrlib>:"Synchronous Latch.vi"("clear"=w616, "set"=w617) -> ("out"=→"Generator On":bool)  [unwired: 9 in]
    n357 = Or(x="Stop Gen App", y=w621) -> (x .or. y?=w613:bool)
    n358 = node-c288() -> ()  [unwired: 1 in, 1 out]
    n359 = Select(t=Generator_States."CloseApp", s=w613, f=w619) -> (s? t:f=w620:T4)
    "Gen State" <- w623
  }
  "Error Out Gen" <- w38
  n360 = timed-loop "Exit App Loop" {
    timing: w11 -> [_]
    timing-out: [_] -> w10
    stop <- w678 stop-if-true
    n361 = node-c288() -> ()  [unwired: 1 in, 1 out]
    n362 = event shown="[1] \"EXIT APP\": Value Change" {
      selector: _ -> [_ _]
      dyn-events: _ -> [_ _]
      timeout: _ -> [_ _]
      tunnel: [_ w686] -> w678
      event Timeout {
        n363 = event-data() -> ()  [unwired: 1 in, 3 out]
      }
      event "EXIT APP": Value Change {
        n364 = event-data() -> ()  [unwired: 1 in, 6 out]
        n365 = flat-sequence {
          tunnel: [w687] -> w685
          tunnel: w685 -> [w690]
          tunnel: [w689] -> w684
          tunnel: w684 -> [w705]
          tunnel: [w704] -> w683
          tunnel: [w703] -> w682
          tunnel: w683 -> [w709]
          tunnel: w682 -> [w707]
          tunnel: [w707] -> w681
          tunnel: ["EXIT APP"] -> w686
          tunnel: w681 -> [w723]
          frame #0 {
            w688 = TRUE ("Stop Gen App")
            n366 = call <vilib>:"Set Busy.vi"() -> ()  [unwired: 10 in, 2 out]
            n367 = local write "Stop Stage App"(w688) -> ()
            n368 = local write "Stop Gen App"(w688) -> ()
            n369 = local write "Stop Digi App"(w688) -> ()
            n370 = local write "Stop File App"(w688) -> ()
            n371 = Tick Count (ms)() -> (millisecond timer value=w687:u32)
          }
          frame #1 {
            n372 = while {
              shift-right: [w697] -> _
              shift-left: w690 -> [w697]
              tunnel: [w691] -> w689
              stop <- w694 stop-if-true
              n373 = local read "Generator On"() -> (w702:bool)
              n374 = local read "File Open?"() -> (w701:bool)
              n375 = local read "Digitizer On"() -> (w700:bool)
              n376 = local read "Controller Open?"() -> (w699:bool)
              n377 = Tick Count (ms)() -> (millisecond timer value=w698:u32)
              n378 = Subtract(x=w698, y=w697) -> (x-y=w696:u32)
              n379 = Greater?(x=w696, y=u32 5000) -> (0:w693:bool)
              n380 = Compound Arithmetic op=OR(w702, w701, w700, w699) -> (invert w692:bool)
              n381 = Or(x=w692, y=w693) -> (x .or. y?=w694:bool)
              n382 = Not(x=w692) -> (.not. x?=w691:bool)
            }
          }
          frame #2 {
            w706 = FALSE ("Stop Gen App")
            n383 = call "Display Message to User"("Enable"=w705) -> ("error out"=w704:errorcluster, "OK"=w703:bool)  [unwired: 9 in]
            n384 = local write "Stop Stage App"(w706) -> ()
            n385 = local write "Stop Gen App"(w706) -> ()
            n386 = local write "Stop Digi App"(w706) -> ()
            n387 = local write "Stop File App"(w706) -> ()
          }
          frame #3 {
            w712 = TRUE ("force destroy? (F)")
            n388 = Obtain Queue(name (unnamed)="AquiredDataFIFOCopy", element data type=T10 {"Wave Count"=0, "Wave"=[]} ("input cluster"), create if not found? (T)=TRUE, error in (no error)=w709) -> (queue out=w714:refnum<queue>, error out=w710:errorcluster)  [unwired: 1 in, 1 out]
            n389 = Obtain Queue(name (unnamed)="AquiredDataFIFO", element data type=T16 {"Wave Count"=0, "Amplitude"=0, "Index"=0} ("cluster"), create if not found? (T)=TRUE, error in (no error)=w710) -> (queue out=w715:refnum<queue>, error out=w711:errorcluster)  [unwired: 1 in, 1 out]
            n390 = Release Queue(queue=w715, force destroy? (F)=w712, error in (no error)=w711) -> (error out=w713:errorcluster)  [unwired: 2 out]
            n391 = Release Queue(queue=w714, force destroy? (F)=w712, error in (no error)=w713) -> ()  [unwired: 3 out]
          }
          frame #4 {
            n392 = control-ref of="This VI"() -> (w724:refnum<vi>)
            n393 = Stop(stop? (T)=w723) -> ()
            n394 = call <vilib>:"Unset Busy.vi"() -> ()  [unwired: 11 in, 1 out]
            n395 = invoke class="VI" method="FP.Close"(reference=w724) -> (reference out=w722:refnum<vi>, error out=w721:errorcluster)  [unwired: 2 in, 1 out]
            n396 = Close Reference(reference=w722, error in (no error)=w721) -> ()  [unwired: 1 out]
          }
        }
      }
    }
    n397 = node-c288() -> ()  [unwired: 1 in, 1 out]
  }
  n398 = disable-structure shown="Disabled" {
    frame Disabled {
      n399 = control-ref of="This VI"() -> (w726:refnum<vi>)
      n400 = call "LoadAllCtrlsConfig.vi"("VI in"=w726) -> ()  [unwired: 11 in]
      n401 = call "StoreAllCtrlsConfig.vi"("VI in"=w726) -> ()  [unwired: 11 in]
    }
    frame Enabled {
    }
  }
  n402 = node-c288(w57) -> ()  [unwired: 1 out]
  n403 = node-c288(w10) -> ()  [unwired: 1 out]
  n404 = node-c288() -> (w2:T18)  [unwired: 2 in]
  n405 = node-c288() -> (w64:T18)  [unwired: 1 in]
  n406 = node-c288() -> (w14:T18)  [unwired: 1 in]
  n407 = Obtain Queue(name (unnamed)="AquiredDataFIFO", element data type=T16 {"Wave Count"=0, "Amplitude"=0, "Index"=0} ("cluster"), create if not found? (T)=TRUE) -> (queue out=w18:refnum<queue>, error out=w17:errorcluster)  [unwired: 2 in, 1 out]
  n408 = Obtain Queue(name (unnamed)="AquiredDataFIFOCopy", element data type=T10 {"Wave Count"=0, "Wave"=[]} ("input cluster"), create if not found? (T)=TRUE, error in (no error)=w17) -> (queue out=w39:refnum<queue>, error out=w40:errorcluster)  [unwired: 1 in, 1 out]
  n409 = Obtain Queue(name (unnamed)="AquiredDataFIFO", element data type=T16 {"Wave Count"=0, "Amplitude"=0, "Index"=0} ("cluster"), create if not found? (T)=TRUE) -> (queue out=w54:refnum<queue>, error out=w53:errorcluster)  [unwired: 2 in, 1 out]
  n410 = Obtain Queue(name (unnamed)="AquiredDataFIFO_Wave", element data type=T10 {"Wave Count"=0, "Wave"=[]} ("input cluster"), create if not found? (T)=TRUE) -> (queue out=w27:refnum<queue>, error out=w28:errorcluster)  [unwired: 2 in, 1 out]
  n411 = while "Image View" {
    shift-right: [w734] -> _
    shift-left: w54 -> [w737]
    shift-right: [w733] -> _
    shift-left: w53 -> [w732]
    tunnel: [w736] -> w3
    tunnel: w12 -> [w728]
    tunnel: w12 -> [w727]
    stop <- w735 stop-if-true
    n412 = call <extravilib>:"Read.vi"("channel"=w736) -> ("element"=w735:bool)  [unwired: 1 in, 1 out]
    n413 = Dequeue Element(queue=w737, timeout in ms (-1)=150, error in (no error)=w732) -> (queue out=w734:refnum<queue>, element=w729:T16, timed out?=w731:bool, error out=w733:errorcluster)
    n414 = case shown="False" w731 {
      tunnel: w729 -> [w748 _]
      tunnel: [w739 _] -> w728
      tunnel: w727 -> [w738 _]
      frame False {
        n415 = local read "Total Pixels"() -> (w745:u64)
        n416 = Unbundle By Name(w748) -> ("Index"=w740:u16, "Amplitude"=w747:i16, "Wave Count"=w746:u64)
        n417 = Increment(x=w746) -> (x+1=w744:u64)
        n418 = Less Or Equal?(x=w744, y=w745) -> (x <= y?=w741:bool)
        n419 = Compound Arithmetic op=AND(w741, "Imaging") -> (w743:bool)
        n420 = case shown="True" w743 {
          selector: w743 -> [w749 _]
          tunnel: w746 -> [_ w759]
          tunnel: w747 -> [_ w753]
          tunnel: w741 -> [_ _]
          tunnel: w740 -> [_ _]
          tunnel: [_ w756] -> w739
          tunnel: w738 -> [_ w755]
          frame False {
            n421 = local write "Imaging"(w749) -> ()
          }
          frame True {
            n422 = local read "Scan Mode"() -> (w758:enum16{"Raster", "Serpentine"})
            n423 = local read "Pixel Count"() -> (w757:u64)
            n424 = call <extravilib>:"Read.vi"("channel"=w755, "timeout in ms (0)"=1) -> ("element"=w754:dbl[])  [unwired: 1 out]
            n425 = call "ImageIndexMap.vi"("Pixel Count"=w757, "Scan Mode"=w758, "Wave Count in"=w759) -> ("Wave Count out"=w751:u64)  [unwired: 8 in]
            n426 = in-place {
              in-place-border: w753 -> [w760]
              n427 = in-place-array #1(w754, w751) -> ()  [unwired: 1 out]
              n428 = in-place-array #1(w760) -> (w752:dbl[])  [unwired: 1 out]
            }
            n429 = call <extravilib>:"Write.vi"("element"=w752) -> ("channel"=w756:T23)  [unwired: 1 out]
          }
        }
      }
      frame True {
      }
    }
  }
  n430 = timed-loop {
    shift-right: [w774] -> w45
    shift-left: w47 -> [w787]
    shift-right: [w786] -> _
    shift-left: _ -> [w785]
    shift-right: [w776] -> _
    shift-left: Digitizer_StatesMain."Idle" -> [w788]
    shift-right: [w782] -> _
    shift-left: w61 -> [w781]
    shift-right: [w772] -> _
    shift-left: w46 -> [w773]
    shift-right: [w770] -> _
    shift-left: w44 -> [w766]
    tunnel: w3 -> [w763]
    shift-right: [w761] -> _
    shift-left: w32 -> [w762]
    timing: w16 -> [_]
    timing-out: [_] -> w15
    stop <- w764 stop-if-true
    n431 = node-c288() -> ()  [unwired: 1 in, 1 out]
    n432 = Equal To 0?(x=w766) -> (x = 0?=→"Wave Count Zero":bool)
    n433 = case shown="\"Init\"" w788 {
      tunnel: w787 -> [w794 w823 w851 w872 w904 w931]
      tunnel: [w794 w803 w844 w856 w892 w929] -> w774
      tunnel: [w798 w815 w834 w857 w896 _] -> w786
      tunnel: w785 -> [w798 _ w836 w868 w898 w930]
      tunnel: [w799 Digitizer_StatesMain."SetParam" ("f") w840 Digitizer_StatesMain."Read" ("f") w900 Digitizer_StatesMain."Idle" ("f")] -> w775
      tunnel: [_ _ w842 _ _ _] -> w783
      tunnel: [w797 _ w838 w869 w899 _] -> w782
      tunnel: w781 -> [w797 _ _ w869 w899 _]
      tunnel: [TRUE _ _ _ _ w928] -> w780
      tunnel: [_ _ _ _ _ w928] -> w765
      tunnel: [w793 w809 w831 w862 w889 w926] -> w772
      tunnel: w773 -> [w793 w808 w831 w862 w890 w926]
      tunnel: [u16 0 ("Wave Count") u16 0 ("Wave Count") w829 w860 w885 u16 0 ("Wave Count")] -> w771
      tunnel: w766 -> [_ _ w830 w860 w882 _]
      tunnel: w762 -> [w791 w806 w826 w859 w881 w924]
      tunnel: [w791 w805 w826 w859 w880 w924] -> w761
      frame "Idle", Default {
        w795 = FALSE ("TIS Configured?")
        n434 = local write "TIS Configured?"(w795) -> ()
        n435 = local write "Configured?"(w795) -> ()
        n436 = Select(t=Digitizer_StatesMain."Init", s="Start Digi", f=Digitizer_StatesMain."Idle") -> (s? t:f=w799:T9)
      }
      frame "Init" {
        n437 = xnode "Open FPGA VI Reference"("error in"=w823, "resource name"="RIO Resource") -> ("FPGA VI Reference Out"=w813:refnum<k20>, "error out"=w822:errorcluster)
        n438 = Type Cast(type=T24 refnum ("FPGA VI Reference Out"), x=w813) -> (*(type *) &x=w812:T24)
        n439 = call "InitDigitizer.vi"("error in"=w822, "FPGA VI Reference In"=w812) -> ("error out"=w817:errorcluster, "range (Vpp)"=→"Range (Vpp)":dbl, "FPGA VI Reference Out"=w818:T24, "TIS Configured?"=→"TIS Configured?":bool, "Configured?"=→"Configured?":bool)  [unwired: 5 in]
        n440 = call "PXITrigReserve-Unreserve.vi"("error in"=w817, "Mode"=enum16{"Reserve", "Unreserve"}."Reserve", "FPGA VI Reference In"=w818) -> ("error out"=w810:errorcluster, "FPGA VI Reference Out"=w815:T24)  [unwired: 7 in]
        n441 = Flush Queue(queue=w808, error in (no error)=w810) -> (queue out=w809:refnum<queue>, error out=w804:errorcluster)  [unwired: 1 out]
        n442 = Flush Queue(queue=w806, error in (no error)=w804) -> (queue out=w805:refnum<queue>, error out=w803:errorcluster)  [unwired: 1 out]
      }
      frame "SetParam" {
        w848 = FALSE  # vi/nGenTrig
        w832 = sgl 5000.0  # ProcessCompletionDelay Factor
        # "Dis-Arm the trigger before seting the parameters! and then Arm Again"
        n443 = local read "Digi Machine Mode"() -> (w837:T8)
        n444 = call "ConfigAquisitionParam.vi"("Requested Samples Per Pixel"="Record Size", "Downsample [0,1,2]"="Time Division", "ProcessCompletionDelay (us)"=w832, "vi/nGenTrig"=w848, "error in"=w851, "AvgCount_powerOf2"="Amplitude \nAveraging", "Delay (us)"="Delay(us)", "FPGA VI Reference In"=w836) -> ("error out"=w846:errorcluster, "Read Size (Host)"=w838:u16, "FPGA VI Reference Out"=w835:T24)  [unwired: 1 in]
        n445 = Equal?(x=w837, y=DigiMachineStates."Scanning Mode") -> (x = y?=w828:bool)
        n446 = Select(t=Digitizer_StatesMain."Read" ("f"), s=w828, f=Digitizer_StatesMain."VITrig") -> (s? t:f=w840:T9)
        n447 = call "Arm(CommitSettings).vi"("Arm?"=TRUE, "error in"=w846, "FPGA VI Reference In"=w835) -> ("error out"=w844:errorcluster, "FPGA VI Reference Out"=w834:T24)  [unwired: 7 in]
        n448 = Unbundle By Name(w844) -> ("status"=w843:bool)
        n449 = Select(t=u16 0, s=w828, f=w830) -> (s? t:f=w829:u64)
        n450 = Not(x=w843) -> (.not. x?=w842:bool)
      }
      frame "VITrig" {
        n451 = Not(x="Pause Triggger") -> (.not. x?=w861:bool)
        n452 = call <instrlib>:"Detect Rising Edge.vi"("signal"="Trigger Digi Single") -> ("edge detected"=w864:bool)  [unwired: 14 in]
        n453 = Equal?(x="Digi Machine Mode", y=DigiMachineStates."Single Shot Mode") -> (x = y?=w866:bool)
        n454 = Select(t=w864, s=w866, f=w861) -> (s? t:f=w863:bool)
        n455 = call "ViTrig.vi"("Vi Trigger"=w863, "error in"=w872, "FPGA VI Reference In"=w868) -> ("error out"=w855:errorcluster, "FPGA VI Reference Out"=w867:T24)  [unwired: 7 in]
        n456 = case shown="True" w861 {
          frame False {
          }
          frame True {
            n457 = Wait (ms)(milliseconds to wait=u32 150) -> ()  [unwired: 1 out]
          }
        }
        n458 = Not Equal?(x="Digi Machine Mode", y=DigiMachineStates."Idle Mode") -> (x != y?=w854:bool)
        n459 = call "Arm(CommitSettings).vi"("Arm?"=w854, "error in"=w855, "FPGA VI Reference In"=w867) -> ("error out"=w856:errorcluster, "FPGA VI Reference Out"=w857:T24)  [unwired: 7 in]
      }
      frame "Read" {
        n460 = call "ReadFromDigi.vi"("Timeout (ms)"=500, "error in"=w904, "Number of Elements"=w899, "FPGA VI Reference In"=w898) -> ("error out"=w895:errorcluster, "Data Valid?"=w884:bool, "Output Waveform"=w893:u16[], "FPGA VI Reference Out"=w897:T24)  [unwired: 4 in]
        n461 = To Word Integer(number=w893) -> (16bit integer=w888:i16[])
        n462 = Bundle By Name(cluster=T10 {"Wave Count"=0, "Wave"=[]} ("input cluster"), "Wave Count"=w882, "Wave"=w888) -> (w886:T10)
        n463 = Increment(x=w882) -> (x+1=w883:u64)
        n464 = call "Arm(CommitSettings).vi"("Arm?"=TRUE, "error in"=w895, "FPGA VI Reference In"=w897) -> ("error out"=w891:errorcluster, "FPGA VI Reference Out"=w896:T24)  [unwired: 7 in]
        n465 = Select(t=w883, s=w884, f=w882) -> (s? t:f=w885:u64)
        n466 = local read "Digi Machine Mode"() -> (w876:T8)
        n467 = Equal?(x=w876, y=DigiMachineStates."Idle Mode") -> (x = y?=w874:bool)
        n468 = Equal?(x=w876, y=DigiMachineStates."Scanning Mode") -> (x = y?=w878:bool)
        n469 = Or(x=w878, y=w874) -> (x .or. y?=w875:bool)
        n470 = case shown="True" w884 {
          tunnel: w886 -> [_ w908]
          tunnel: w891 -> [w907 w910]
          tunnel: [w907 w911] -> w892
          tunnel: w890 -> [w906 w916]
          tunnel: [w906 w915] -> w889
          tunnel: w881 -> [w905 w914]
          tunnel: [w905 w913] -> w880
          tunnel: w875 -> [_ w909]
          frame False {
          }
          frame True {
            n471 = Enqueue Element(queue=w916, element=w908, error in (no error)=w910) -> (queue out=w915:refnum<queue>, error out=w912:errorcluster)  [unwired: 1 in, 1 out]
            n472 = case shown="False" w909 {
              tunnel: w914 -> [w921 w923]
              tunnel: [w920 w923] -> w913
              tunnel: w912 -> [w919 w922]
              tunnel: [w918 w922] -> w911
              tunnel: w908 -> [w917 _]
              frame False {
                n473 = Enqueue Element(queue=w921, element=w917, error in (no error)=w919) -> (queue out=w920:refnum<queue>, error out=w918:errorcluster)  [unwired: 1 in, 1 out]
              }
              frame True {
              }
            }
            "Wave out packet" <- w908
          }
        }
        n474 = Select(t=Digitizer_StatesMain."Read" ("f"), s=w878, f=Digitizer_StatesMain."SetParam") -> (s? t:f=w900:T9)
      }
      frame "CloseApp" {
        w928 = TRUE
        n475 = call "PXITrigReserve-Unreserve.vi"("error in"=w931, "Mode"=enum16{"Reserve", "Unreserve"}."Unreserve", "FPGA VI Reference In"=w930) -> ("error out"=w932:errorcluster, "FPGA VI Reference Out"=w933:T24)  [unwired: 7 in]
        n476 = xnode "Close FPGA VI Reference"("FPGA VI Reference In"=w933, "error in"=w932) -> ("error out"=w929:errorcluster)
      }
    }
    n477 = call <vilib>:"Share Stop Signal.vi"("set stop (F)"=w765, "channel"=w763) -> ("stop"=w764:bool)
    "nDigiLoopRunning" <- w764
    n478 = call <instrlib>:"Synchronous Latch.vi"("clear"=w780, "set"=w783) -> ("out"=→"Digitizer On":bool)  [unwired: 9 in]
    n479 = Or(x="Stop Digi App", y=w774) -> (x .or. y?=w778:bool)
    n480 = Select(t=u64 0, s="CountReset", f=w771) -> (s? t:f=w770:u64)
    n481 = node-c288() -> ()  [unwired: 1 in, 1 out]
    n482 = Select(t=Digitizer_StatesMain."CloseApp", s=w778, f=w775) -> (s? t:f=w776:T9)
    "Digi State" <- w788
  }
  "error out Digi" <- w45
  n483 = timed-loop "Change Digitizer Mode" {
    timing: w37 -> [_]
    timing-out: [_] -> w36
    tunnel: w3 -> [w935]
    stop <- w936 stop-if-true
    n484 = node-c288() -> ()  [unwired: 1 in, 1 out]
    n485 = event shown="[0] Timeout" {
      selector: _ -> [_ _ _ _ _ _]
      dyn-events: _ -> [_ _ _ _ _ _]
      timeout: 0 -> [_ _ _ _ _ _]
      event Timeout {
        w938 = FALSE ("Start Digi")
        n486 = event-data() -> ()  [unwired: 1 in, 3 out]
        n487 = local read "Digi Machine Mode"() -> (w939:T8)
        n488 = local write "Trigger Digi Single"(w938) -> ()
        n489 = local write "Start Digi"(w938) -> ()
        n490 = case shown="\"Idle Mode\"" w939 {
          frame "Live Mode" {
            w940 = FALSE ("Value (Signaling)")
            n491 = Not(x=w940) -> (.not. x?=w941:bool)
            n492 = local write "Single Shot"(w940) -> ()
            n493 = local write "Scanning"(w940) -> ()
            n494 = local write "LIVE"(w941) -> ()
          }
          frame "Single Shot Mode" {
            w943 = FALSE ("Value (Signaling)")
            n495 = Not(x=w943) -> (.not. x?=w942:bool)
            n496 = local write "Single Shot"(w942) -> ()
            n497 = local write "Scanning"(w943) -> ()
            n498 = local write "LIVE"(w943) -> ()
          }
          frame "Scanning Mode" {
            w945 = FALSE ("Value (Signaling)")
            n499 = Not(x=w945) -> (.not. x?=w944:bool)
            n500 = local write "Single Shot"(w945) -> ()
            n501 = local write "Scanning"(w944) -> ()
            n502 = local write "LIVE"(w945) -> ()
          }
          frame "Idle Mode" {
            w946 = FALSE ("Value (Signaling)")
            n503 = local write "LIVE"(w946) -> ()
            n504 = local write "Single Shot"(w946) -> ()
            n505 = local write "Scanning"(w946) -> ()
          }
        }
      }
      event "TriggerDigi": Value Change {
        n506 = event-data() -> ()  [unwired: 1 in, 6 out]
        n507 = local write "Trigger Digi Single"(TRUE ("Trigger Digi Single")) -> ()
      }
      event "LIVE": Value Change {
        n508 = event-data() -> ()  [unwired: 1 in, 6 out]
        n509 = local write "Digi Machine Mode"(DigiMachineStates."Live Mode" ("Digi Machine Mode")) -> ()
      }
      event "Single Shot": Value Change {
        n510 = event-data() -> ()  [unwired: 1 in, 6 out]
        n511 = local write "Digi Machine Mode"(DigiMachineStates."Single Shot Mode" ("Digi Machine Mode")) -> ()
      }
      event "Scanning": Value Change {
        n512 = event-data() -> ()  [unwired: 1 in, 6 out]
        n513 = local write "Digi Machine Mode"(DigiMachineStates."Scanning Mode" ("Digi Machine Mode")) -> ()
      }
      event "Start Digitizer UI Bttn": Value Change {
        n514 = event-data() -> ()  [unwired: 1 in, 6 out]
        n515 = local write "Start Digi"(TRUE ("Start Digi")) -> ()
      }
    }
    n516 = node-c288() -> ()  [unwired: 1 in, 1 out]
    n517 = call <extravilib>:"Read.vi"("channel"=w935) -> ("element"=w936:bool)  [unwired: 1 in, 1 out]
  }
  n518 = while "Save Image" {
    tunnel: w3 -> [w955]
    stop <- w954 stop-if-true
    n519 = event shown="[0] \"Save Img\": Value Change" {
      selector: _ -> [_ _]
      dyn-events: _ -> [_ _]
      timeout: 500 -> [_ _]
      event "Save Img": Value Change {
        n520 = event-data() -> ("NewVal"=w957:bool)  [unwired: 1 in, 5 out]
        n521 = case shown="True" w957 {
          frame False {
          }
          frame True {
            w963 = 24
            # "SAVE INTENSITY GRAPH"
            n522 = control-ref of="Image Display"() -> (w960:refnum<vi>)
            n523 = invoke class="IntGraph (strict)" method="Get Image"(reference=w960, "image depth"=w963) -> (reference out=w958:refnum<vi>, error out=w959:errorcluster, "image data"=w977:T25)  [unwired: 4 in, 3 out]
            n524 = local read "FilenameSimeStamped"() -> (w962:string)
            n525 = local read "FileDirectoryFinal"() -> (w961:path)
            n526 = disable-structure shown="Disabled" {
              disable-tunnel: [w989 _] -> w971
              disable-tunnel: w963 -> [w984 _]
              disable-tunnel: w962 -> [w983 _]
              disable-tunnel: w961 -> [w982 _]
              frame Disabled {
                n527 = control-ref of="Topography Plot"() -> (w981:refnum<vi>)
                n528 = invoke class="LabVIEW 3D Graph (strict)" method="Get Image"(reference=w981, "image depth"=w984) -> (reference out=w980:refnum<vi>, error out=w979:errorcluster, "image data"=w990:T25)  [unwired: 4 in, 3 out]
                n529 = Close Reference(reference=w980, error in (no error)=w979) -> ()  [unwired: 1 out]
                n530 = Concatenate Strings(w983, "-Index.jpeg" ("string")) -> (w986:string)
                n531 = String To Path(string=w986) -> (path=w985:path)
                n532 = Build Path(base path=w982, name or relative path=w985) -> (appended path=w988:path)
                n533 = call <vilib>:"Write JPEG File.vi"("quality (80)"=100, "image data"=w990, "path to JPEG file"=w988) -> ("error out"=w989:errorcluster)  [unwired: 7 in, 1 out]
              }
              frame Enabled {
              }
            }
            n534 = Close Reference(reference=w958, error in (no error)=w959) -> ()  [unwired: 1 out]
            n535 = Concatenate Strings(w962, "-Amplitudes.jpeg" ("string")) -> (w968:string)
            n536 = String To Path(string=w968) -> (path=w969:path)
            n537 = Build Path(base path=w961, name or relative path=w969) -> (appended path=w970:path)
            n538 = call <vilib>:"Write JPEG File.vi"("quality (80)"=100, "image data"=w977, "path to JPEG file"=w970) -> ("error out"=w975:errorcluster)  [unwired: 7 in, 1 out]
            n539 = Merge Errors(w975, w971) -> (w965:errorcluster)
            n540 = Unbundle By Name(w965) -> ("status"=w966:bool)
            n541 = call <vilib>:"Clear Errors.vi"("error in (no error)"=w965, "specific error code to clear (0: all)"=43) -> ("error out"=w973:errorcluster, "specific error cleared?"=w974:bool)  [unwired: 4 in]
            n542 = Not(x=w966) -> (.not. x?=w964:bool)
            n543 = call "Display Message to User2"("error in (no error)"=w973, "Enable"=w974) -> ("error out"=w972:errorcluster)  [unwired: 8 in, 1 out]
            n544 = call "Display Message to User3"("Enable"=w964) -> ()  [unwired: 9 in, 2 out]
            n545 = call <vilib>:"Clear Errors.vi"("error in (no error)"=w972) -> ()  [unwired: 5 in, 2 out]
          }
        }
      }
      event Timeout {
        n546 = event-data() -> ()  [unwired: 1 in, 3 out]
      }
    }
    n547 = call <extravilib>:"Read.vi"("channel"=w955) -> ("element"=w954:bool)  [unwired: 1 in, 1 out]
  }
  n548 = node-c288(w36) -> ()  [unwired: 1 out]
  n549 = node-c288(w15) -> ()  [unwired: 1 out]
  n550 = timed-loop "Z Axis Control Loop" {
    tunnel: w3 -> [w1009]
    shift-right: [w994] -> _
    shift-left: Z_Axis_States."Init" -> [w1008]
    shift-right: [w1005] -> _
    shift-left: errorcluster {"status"=FALSE, "code"=0, "source"=""} ("error out") -> [w1006]
    shift-right: [w1004] -> _
    shift-left: w7 -> [w1002]
    shift-right: [w1003] -> _
    shift-left: w6 -> [w1001]
    timing: w2 -> [_]
    timing-out: [_] -> w1
    stop <- w995 stop-if-true
    n551 = node-c288() -> ()  [unwired: 1 in, 1 out]
    n552 = case shown="\"cmd_MoveDown Rel\"" w1008 {
      tunnel: [w1015 Z_Axis_States."Idle" Z_Axis_States."Idle" Z_Axis_States."Idle" Z_Axis_States."Idle" Z_Axis_States."Idle" Z_Axis_States."Idle" Z_Axis_States."Idle"] -> w1007
      tunnel: [_ w1026 _ _ _ _ _ _] -> w1000
      tunnel: w1006 -> [w1012 w1030 w1041 w1051 w1063 w1075 w1083 w1090]
      tunnel: [w1012 w1024 w1033 w1044 w1055 w1072 w1080 w1087] -> w1005
      tunnel: [w1014 w1028 w1037 w1047 w1056 w1070 T15 refnum ("KCubeServoControl out") w1085] -> w1004
      tunnel: [w1013 w1027 w1038 w1048 w1057 w1071 w1079 w1086] -> w1003
      tunnel: w1002 -> [w1014 _ w1039 w1049 w1065 w1073 w1081 w1088]
      tunnel: w1001 -> [w1013 _ w1040 w1050 w1064 w1074 w1082 w1089]
      tunnel: [_ w1023 w1032 w1043 w1060 _ w1076 _] -> w998
      tunnel: "Z Step (mm)" -> [_ _ w1036 w1046 _ _ _ _]
      tunnel: "Z_Speed (mm/s)" -> [_ _ _ _ _ w1067 _ _]
      tunnel: [_ w1022 _ _ _ _ w1076 _] -> w995
      frame "Idle", Default {
        n553 = event shown="[0] Timeout" {
          selector: _ -> [_ _ _ _ _]
          dyn-events: _ -> [_ _ _ _ _]
          timeout: 200 -> [_ _ _ _ _]
          tunnel: [Z_Axis_States."cmd_GetPos" Z_Axis_States."cmd_MoveUp Rel" Z_Axis_States."cmd_MoveDown Rel" Z_Axis_States."cmd_SetVel" Z_Axis_States."cmd_stop"] -> w1015
          event Timeout {
            n554 = event-data() -> ()  [unwired: 1 in, 3 out]
          }
          event "Z_Move Up": Value Change {
            n555 = event-data() -> ()  [unwired: 1 in, 6 out]
          }
          event "Z_MoveDown": Value Change {
            n556 = event-data() -> ()  [unwired: 1 in, 6 out]
          }
          event "Z_Speed (mm/s)": Value Change {
            n557 = event-data() -> ()  [unwired: 1 in, 6 out]
          }
          event "Z_Stop": Value Change {
            n558 = event-data() -> ()  [unwired: 1 in, 6 out]
          }
        }
      }
      frame "Init" {
        n559 = call <vilib>:"Set Busy.vi"("error in (no error)"=w1030) -> ("error out"=w1025:errorcluster)  [unwired: 9 in, 1 out]
        n560 = call "Thor_OpenDevice.vi"("error in (no error)"=w1025) -> ("error out"=w1029:errorcluster, "Device"=w1027:T14, "KCubeServoControl out"=w1028:T15, "CreateDevice?"=w1026:bool)  [unwired: 7 in]
        n561 = call <vilib>:"Unset Busy.vi"("error in (no error)"=w1029) -> ("error out"=w1024:errorcluster)  [unwired: 10 in]
        n562 = Not(x=w1026) -> (.not. x?=w1023:bool)
        n563 = call "Display Message to User4"("Enable"=w1023) -> ("OK"=w1022:bool)  [unwired: 9 in, 1 out]
      }
      frame "cmd_MoveUp Rel" {
        w1035 = 2 items=["Forward"=1, "Backward"=2] ("Direction")
        n564 = call "Thor_MoveRelative.vi"("Step Size"=w1036, "Direction"=w1035, "error in"=w1041, "Device In"=w1040, "KCubeServoControl In"=w1039) -> ("error out"=w1033:errorcluster, "Device Out"=w1038:T14, "KCubeServoControl out"=w1037:T15)  [unwired: 4 in]
        n565 = Unbundle By Name(w1033) -> ("status"=w1032:bool)
      }
      frame "cmd_MoveDown Rel" {
        w1045 = 1 items=["Forward"=1, "Backward"=2] ("Direction")
        n566 = call "Thor_MoveRelative.vi"("Step Size"=w1046, "Direction"=w1045, "error in"=w1051, "Device In"=w1050, "KCubeServoControl In"=w1049) -> ("error out"=w1044:errorcluster, "Device Out"=w1048:T14, "KCubeServoControl out"=w1047:T15)  [unwired: 4 in]
        n567 = Unbundle By Name(w1044) -> ("status"=w1043:bool)
      }
      frame "cmd_GetPos" {
        n568 = call "Thor_GetPosition.vi"("error in"=w1063, "Device In"=w1064, "KCubeServoControl In"=w1065) -> ("error out"=w1059:errorcluster, "Position"=→"Z (mm)":dbl, "Device Out"=w1058:T14, "KCubeServoControl out"=w1054:T15)  [unwired: 5 in]
        n569 = call "Thor_GetStatus.vi"("error in (no error)"=w1059, "Device In"=w1058, "KCubeServoControl In"=w1054) -> ("error out"=w1055:errorcluster, "Device Out"=w1057:T14, "KCubeServoControl out"=w1056:T15, "Z Moving?"=→"Z Moving?":bool, "HW LimitSwitches"=→"At Limit":bool)  [unwired: 4 in]
        n570 = Unbundle By Name(w1055) -> ("status"=w1060:bool)
      }
      frame "cmd_SetVel" {
        n571 = call "Thor_GetSEtVelParam.vi"("acceleration"=0.5, "maxVelocity"=w1067, "error in (no error)"=w1075, "Set Param"=TRUE, "Device In"=w1074, "KCubeServoControl In"=w1073) -> ("error out"=w1072:errorcluster, "Device Out"=w1071:T14, "KCubeServoControl out"=w1070:T15)  [unwired: 1 in, 2 out]
      }
      frame "Close Z" {
        w1076 = TRUE ("status")
        n572 = call "Thor_CloseDevice.vi"("error in (no error)"=w1083, "Device In"=w1082, "KCubeServoControl In"=w1081) -> ("error out"=w1080:errorcluster, "Device Out"=w1079:T14)  [unwired: 6 in, 1 out]
      }
      frame "cmd_stop" {
        n573 = call "Thor_StopImmidiate.vi"("error in (no error)"=w1090, "Device In"=w1089, "KCubeServoControl In"=w1088) -> ("error out"=w1087:errorcluster, "Device Out"=w1086:T14, "KCubeServoControl out"=w1085:T15)  [unwired: 6 in]
      }
    }
    n574 = call <instrlib>:"Synchronous Latch.vi"("clear"=w998, "set"=w1000) -> ("out"=→"Z Open?":bool)  [unwired: 9 in]
    n575 = call <extravilib>:"Read.vi"("channel"=w1009) -> ("element"=w993:bool)  [unwired: 1 in, 1 out]
    n576 = node-c288() -> ()  [unwired: 1 in, 1 out]
    n577 = Select(t=Z_Axis_States."Close Z", s=w993, f=w1007) -> (s? t:f=w994:T7)
    "Z Axis State" <- w1008
  }
  n578 = timed-loop "Digitizer UI Handle" {
    timing: w64 -> [_]
    timing-out: [_] -> w63
    tunnel: w3 -> [w1092]
    stop <- w1091 stop-if-true
    n579 = First Call?() -> (First Call?: T/F=w1093:bool)
    n580 = node-c288() -> ()  [unwired: 1 in, 1 out]
    n581 = call <extravilib>:"Read.vi"("channel"=w1092) -> ("element"=w1091:bool)  [unwired: 1 in, 1 out]
    n582 = case shown="True" w1093 {
      frame False {
      }
      frame True {
        n583 = property on="Delay(us)" class="DigNum (strict)"("Val(Sgnl)"=sgl 0.0 ("Value (Signaling)")) -> ()  [unwired: 2 in, 2 out]
      }
    }
    n584 = event shown="[1] \"Amplitude Range\": Value Change" {
      selector: _ -> [_ _ _ _]
      dyn-events: _ -> [_ _ _ _]
      timeout: 0 -> [_ _ _ _]
      event Timeout {
        n585 = event-data() -> ()  [unwired: 1 in, 3 out]
      }
      event "Amplitude Range": Value Change {
        n586 = event-data() -> ("NewVal"=w1101:cluster{"Slider 1":dbl, "Slider 1":dbl})  [unwired: 1 in, 5 out]
        n587 = Unbundle(w1101) -> ("Slider 1"=w1100:dbl, "Slider 1"=w1099:dbl)
        n588 = Less?(x=w1100, y=w1099) -> (x < y?=w1098:bool)
        n589 = case shown="True" w1098 {
          tunnel: w1100 -> [_ w1103]
          tunnel: w1099 -> [_ w1102]
          frame False {
          }
          frame True {
            n590 = property on="Waveform [LIVE]" class="WFGraph (strict)"("YScale.Minimum"=w1103, "YScale.Maximum"=w1102) -> ()  [unwired: 2 in, 2 out]
          }
        }
      }
      event "FineDelayControl": Value Change {
        n591 = event-data() -> ("OldVal"=w1107:dbl, "NewVal"=w1108:dbl)  [unwired: 1 in, 4 out]
        n592 = Subtract(x=w1108, y=w1107) -> (x-y=w1106:dbl)
        n593 = property on="Delay(us)" class="DigNum (strict)"() -> ("Value"=w1105:sgl)  [unwired: 2 in, 2 out]
        n594 = Add(x=w1106, y=w1105) -> (x+y=w1104:dbl)
        n595 = property on="Delay(us)" class="DigNum (strict)"("Value"=w1104) -> ()  [unwired: 2 in, 2 out]
      }
      event "Delay_Scroll_Range", "Delay(us)": Value Change {
        w1111 = 0.1 ("Scale.Range:Increment")
        n596 = event-data() -> ()  [unwired: 1 in, 6 out]
        n597 = property on="Delay(us)" class="DigNum (strict)"() -> ("Value"=w1109:sgl)  [unwired: 2 in, 2 out]
        n598 = Subtract(x=w1109, y="Delay_Scroll_Range") -> (x-y=w1113:dbl)
        n599 = Add(x=w1109, y="Delay_Scroll_Range") -> (x+y=w1112:dbl)
        n600 = property on="FineDelayControl" class="Slide (strict)"("Scale.Increment"=w1111, "Scale.MinorInc"=w1111, "Scale.Minimum"=w1113, "Scale.Maximum"=w1112, "Value"=w1109) -> ()  [unwired: 2 in, 2 out]
      }
    }
    n601 = node-c288() -> ()  [unwired: 1 in, 1 out]
  }
  n602 = while "File I/O Loop" {
    shift-right: [w1120] -> _
    shift-left: Data_Save_State."Idle" -> [w1133]
    shift-right: [w1114] -> w23
    shift-left: w40 -> [w1126]
    shift-right: [w1125] -> _
    shift-left: w51 -> [w1123]
    shift-right: [w1124] -> _
    shift-left: w50 -> [w1122]
    shift-right: [w1118] -> _
    shift-left: w39 -> [w1119]
    shift-right: [w1116] -> _
    shift-left: w18 -> [w1117]
    stop <- w1121 stop-if-true
    n603 = case shown="\"Idle\", Default" w1133 {
      tunnel: [w1138 Data_Save_State."Write Attributes" Data_Save_State."Append Data" w1213 Data_Save_State."Idle" Data_Save_State."Idle"] -> w1132
      tunnel: [TRUE ("Ext/nViTrig") _ _ _ TRUE ("Ext/nViTrig") w1259] -> w1128
      tunnel: [_ _ _ _ _ w1259] -> w1121
      tunnel: [_ _ TRUE ("Elements Added?") TRUE ("Elements Added?") _ _] -> w1127
      tunnel: w1126 -> [w1145 w1156 w1190 w1204 w1252 w1263]
      tunnel: [w1145 w1155 w1189 w1200 w1251 w1262] -> w1114
      tunnel: [w1143 w1154 w1188 w1208 w1248 w1258] -> w1125
      tunnel: [w1144 w1153 w1187 w1209 w1247 w1257] -> w1124
      tunnel: w1123 -> [w1143 _ w1191 w1208 w1250 w1261]
      tunnel: w1122 -> [w1144 _ w1187 w1210 w1249 w1260]
      tunnel: w1119 -> [w1142 w1150 w1160 w1206 w1245 w1255]
      tunnel: [w1142 w1150 w1160 w1196 w1245 w1255] -> w1118
      tunnel: w1117 -> [w1136 w1147 w1158 w1201 w1244 w1254]
      tunnel: [w1136 w1147 w1158 w1199 w1244 w1254] -> w1116
      frame "Idle", Default {
        n604 = Select(t=Data_Save_State."Open File", s="Open File", f=Data_Save_State."Idle") -> (s? t:f=w1146:T11)
        n605 = Select(t=Data_Save_State."Close File", s="Done Recording", f=w1146) -> (s? t:f=w1138:T11)
      }
      frame "Open File" {
        n606 = call "H5_RefOpen.vi"("error in (no error)"=w1156, "Filename"="FileName", "File Directory"="File Store Directory") -> ("error out"=w1155:errorcluster, "HDF5 Dataset Ref out"=w1153:T17, "HDF5 Ref out"=w1154:T17, "FilenameSimeStamped"=→"FilenameSimeStamped":string, "FileDirectoryFinal"=→"FileDirectoryFinal":path)  [unwired: 4 in]
      }
      frame "Write Attributes" {
        n607 = local read "Time Division"() -> (w1177:u8)
        n608 = local read "Sampling Frequency (Hz)"() -> (w1175:u64)
        n609 = local read "Speed Control (mm/s)"() -> (w1181:sgl)
        n610 = local read "Scan Time (Approx.)"() -> (w1168:string)
        n611 = Power Of 2(x=w1177) -> (2^x=w1178:dbl)
        n612 = local read "Waves per Pixel"() -> (w1171:u32)
        n613 = local read "Y Step Size (R)"() -> (w1166:sgl)
        n614 = local read "X Step Size (R)"() -> (w1167:sgl)
        n615 = local read "Amplitudes"() -> (w1173:dbl[])
        n616 = local read "Offset Factor"() -> (w1172:dbl)
        n617 = local read "Pixel Count"() -> (w1180:u64)
        n618 = local read "Record Size"() -> (w1169:u16)
        n619 = local read "Scan Mode"() -> (w1182:enum16{"Raster", "Serpentine"})
        n620 = local read "Line Count"() -> (w1179:u64)
        n621 = local read "Delay(us)"() -> (w1165:sgl)
        n622 = Divide(x=1600000000.0 ("Sample Rate"), y=w1178) -> (x/y=w1170:dbl)
        n623 = local read "X Start"() -> (w1186:sgl)
        n624 = local read "Y Start"() -> (w1184:sgl)
        n625 = local read "X End"() -> (w1185:sgl)
        n626 = local read "Y End"() -> (w1183:sgl)
        n627 = local read "Gain"() -> (w1174:dbl)
        n628 = call "H5_WriteAttr.vi"("HDF5 Ref In"=w1191, "X Start"=w1186, "X End"=w1185, "Y Start"=w1184, "Y End"=w1183, "Scan Mode"=w1182, "Speed Control (mm/s)"=w1181, "error in (no error)"=w1190, "Scan Time (Approx.)"=w1168, "Pixel Count"=w1180, "X Step Size (R)"=w1167, "Line Count"=w1179, "Y Step Size (R)"=w1166, "Gen Sampling Rate"=w1175, "Amplitudes (V)"=w1173, "Offset"=w1172, "Gain"=w1174, "Waves per Pixel"=w1171, "Record Size"=w1169, "Delay(us)"=w1165, "Sampling Freq (Hz)"=w1170, "Temperature"="Temperature (C)", "Remarks"="Remarks", "Transducer Freq(Hz)"="Transducer Freq (Hz)", "Immersion Medium"="Immersion Medium") -> ("HDF5 Ref Out"=w1188:T17, "error out"=w1189:errorcluster)  [unwired: 1 in]
      }
      frame "Append Data" {
        n629 = Dequeue Element(queue=w1206, timeout in ms (-1)=150, error in (no error)=w1204) -> (queue out=w1197:refnum<queue>, element=w1205:T10, timed out?=w1198:bool, error out=w1203:errorcluster)
        n630 = case shown="False" w1198 {
          tunnel: w1210 -> [w1238 w1243]
          tunnel: [w1237 w1243] -> w1209
          tunnel: w1205 -> [w1236 _]
          tunnel: w1203 -> [w1235 w1240]
          tunnel: w1201 -> [w1233 w1241]
          tunnel: [w1231 w1240] -> w1200
          tunnel: [w1230 w1241] -> w1199
          tunnel: w1197 -> [w1224 w1242]
          tunnel: [w1224 w1242] -> w1196
          tunnel: [w1218 FALSE] -> w1195
          frame False {
            n631 = Unbundle By Name(w1236) -> ("Wave"=w1217:i16[], "Wave Count"=w1234:u64)
            n632 = Absolute Value(x=w1217) -> (abs(x)=w1216:i16[])
            n633 = call "AppendWaveToFile.vi"("Waveform"=w1217, "error in (no error)"=w1235, "Append?"="Record Data", "HDF5 Dataset Ref"=w1238) -> ("error out"=w1232:errorcluster, "HDF5 Dataset out"=w1237:T17)  [unwired: 5 in, 1 out]
            n634 = Array Max & Min(array=w1216) -> (max value=w1227:i16, max index (indices)=w1228:i32)  [unwired: 2 out]
            n635 = Bundle(cluster=T16 {"Wave Count"=0, "Amplitude"=0, "Index"=0}, "Wave Count"=w1234, "Amplitude"=w1227, "Index"=w1228) -> (w1226:T16)
            n636 = Increment(x=w1234) -> (x+1=w1219:u64)
            n637 = local read "Total Pixels"() -> (w1220:u64)
            n638 = local read "total time (sec)"() -> (w1223:sgl)
            n639 = Enqueue Element(queue=w1233, element=w1226, error in (no error)=w1232) -> (queue out=w1230:refnum<queue>, error out=w1231:errorcluster)  [unwired: 1 in, 1 out]
            n640 = call "FindProgress.vi"("total time (sec)"=w1223, "Total Pixels"=w1220, "Wave Count"=w1219) -> ("TimeString"=→"RemainingTimeString":string, "Progress%"=→"ProgressBar":u8)  [unwired: 7 in]
            n641 = Greater Or Equal?(x=w1219, y=w1220) -> (x >= y?=w1218:bool)
          }
          frame True {
          }
        }
        "No Trig Miss" <- w1195
        n642 = local read "Done Recording"() -> (w1193:bool)
        n643 = Or(x=w1193, y=w1195) -> (x .or. y?=w1194:bool)
        n644 = case shown="True" w1194 {
          frame False {
          }
          frame True {
            n645 = flat-sequence {
              frame #0 {
                n646 = property on="Save Img" class="Bool (strict)"("Val(Sgnl)"=TRUE ("Value (Signaling)")) -> ()  [unwired: 2 in, 2 out]
              }
              frame #1 {
                n647 = property on="Save Img" class="Bool (strict)"("Value"=FALSE ("Value (Signaling)")) -> ()  [unwired: 2 in, 2 out]
              }
            }
          }
        }
        n648 = Select(t=Data_Save_State."Close File", s=w1194, f=Data_Save_State."Append Data") -> (s? t:f=w1213:T11)
      }
      frame "Close File" {
        w1247 = T17 refnum items=["HDF5 Ref"] ("HDF5 Dataset out")
        w1248 = T17 refnum items=["HDF5 Ref"] ("HDF5 Ref out")
        n649 = call "H5_CloseFile.vi"("error in (no error)"=w1252, "HDF5 Dataset Ref"=w1249, "HDF5 Ref"=w1250) -> ("error out"=w1251:errorcluster)  [unwired: 8 in]
      }
      frame "Close App" {
        w1257 = T17 refnum items=["HDF5 Ref"] ("HDF5 Dataset out")
        w1258 = T17 refnum items=["HDF5 Ref"] ("HDF5 Ref out")
        w1259 = TRUE ("Ext/nViTrig")
        n650 = call "H5_CloseFile.vi"("error in (no error)"=w1263, "HDF5 Dataset Ref"=w1260, "HDF5 Ref"=w1261) -> ("error out"=w1262:errorcluster)  [unwired: 8 in]
      }
    }
    n651 = call <instrlib>:"Synchronous Latch.vi"("clear"=w1128, "set"=w1127) -> ("out"=→"File Open?":bool)  [unwired: 9 in]
    n652 = Or(x="Stop File App", y=w1114) -> (x .or. y?=w1115:bool)
    n653 = Select(t=Data_Save_State."Close App" ("f"), s=w1115, f=w1132) -> (s? t:f=w1120:T11)
    "FileStore State" <- w1133
  }
  "Error Out FileIO" <- w23
  n654 = while "Wave View" {
    shift-right: [w1269] -> _
    shift-left: w27 -> [w1272]
    shift-right: [w1268] -> _
    shift-left: w28 -> [w1267]
    tunnel: w3 -> [w1271]
    stop <- w1270 stop-if-true
    n655 = call <extravilib>:"Read.vi"("channel"=w1271) -> ("element"=w1270:bool)  [unwired: 1 in, 1 out]
    n656 = Dequeue Element(queue=w1272, timeout in ms (-1)=150, error in (no error)=w1267) -> (queue out=w1269:refnum<queue>, element=w1264:T10, timed out?=w1266:bool, error out=w1268:errorcluster)
    n657 = case shown="False" w1266 {
      tunnel: w1264 -> [w1276 _]
      frame False {
        n658 = Unbundle By Name(w1276) -> ("Wave"=w1275:i16[], "Wave Count"=→"Waves Count":u64)
        n659 = flat-sequence {
          tunnel: w1275 -> [w1289]
          tunnel: [w1277] -> w1273
          tunnel: w1273 -> [w1290]
          frame #0 {
            n660 = local read "Time Division"() -> (w1287:u8)
            n661 = control-ref of="Waveform [LIVE]"() -> (w1277:refnum<vi>)
            n662 = local read "Range (Vpp)"() -> (w1281:dbl)
            n663 = local read "Delay(us)"() -> (w1283:sgl)
            n664 = Power Of 2(x=w1287) -> (2^x=w1286:dbl)
            n665 = Divide(x=1600000000.0 ("Sample Rate"), y=w1286) -> (x/y=w1285:dbl)
            n666 = call "Scale Acquired Data.vi"("range (V)"=w1281, "Start Time (us)"=w1283, "Sample Rate"=w1285, "Number of Bits"=i16 16, "Data In"=w1289) -> ("output waveform"=w1282:cluster{"Start Time":dbl, dbl, ext[]})  [unwired: 6 out]
            n667 = call "ShowMinMaxOn Graoh.vi"("Log Mode?"="LogMode", "WaveformGraph in"=w1277, "Range (Vpp)"=w1281, "output waveform"=w1282) -> ("Time (sec)"=→"Max Index (s)":dbl, "Max Abs"=→"Max Val (V)":ext)  [unwired: 4 in, 2 out]
          }
          frame #1 {
            n668 = Close Reference(reference=w1290) -> ()  [unwired: 1 in, 1 out]
          }
        }
      }
      frame True {
      }
    }
  }
  n669 = while "LongShot Loop" {
    shift-right: [w1301] -> _
    shift-left: LongShotStates."Idle" -> [w1302]
    shift-right: [w1299] -> _
    shift-left: u8 0 ("Time Division") -> [w1300]
    shift-right: [w1298] -> _
    shift-left: _ -> [w1297]
    shift-right: [w1296] -> _
    shift-left: _ -> [w1295]
    shift-right: [w1294] -> _
    shift-left: _ -> [w1293]
    tunnel: w3 -> [w1292]
    stop <- w1291 stop-if-true
    n670 = case shown="\"Show Data\"" w1302 {
      tunnel: [w1303 w1314 LongShotStates."Clear Wave Count" ("f") w1344 LongShotStates."Set Param" ("f") LongShotStates."Take Shot" ("f") w1387 w1403 LongShotStates."Idle" ("f")] -> w1301
      tunnel: [u8 0 ("Time Division") u8 0 ("Time Division") u8 0 ("Time Division") u8 0 ("Time Division") u8 0 ("Time Division") w1362 w1389 w1391 u8 0 ("Time Division")] -> w1299
      tunnel: w1300 -> [_ _ _ _ _ w1362 w1389 w1396 _]
      tunnel: [_ _ _ _ _ w1359 w1379 _ _] -> w1298
      tunnel: w1297 -> [_ _ _ _ _ _ w1379 _ _]
      tunnel: [_ _ _ _ _ _ w1383 _ _] -> w1296
      tunnel: w1295 -> [_ _ _ _ _ _ _ w1399 _]
      tunnel: [i16[] [] i16[] [] i16[] [] i16[] [] i16[] [] w1361 w1382 w1398 i16[] []] -> w1294
      tunnel: w1293 -> [_ _ _ _ _ w1361 w1382 w1397 w1405]
      frame "Idle", Default {
        n671 = Select(t=LongShotStates."Start Gen", s="LongShot", f=LongShotStates."Idle") -> (s? t:f=w1303:T13)
      }
      frame "Start Gen" {
        # "Start Generator"
        n672 = control-ref of="stop Gen"() -> (w1318:refnum<vi>)
        n673 = control-ref of="Generator On"() -> (w1316:refnum<vi>)
        n674 = control-ref of="Start Gen"() -> (w1317:refnum<vi>)
        n675 = call "SwitchTillOn.vi"("Stop if On?"=TRUE, "Turn Off Button"=w1318, "timeout"=u32 300000, "Turn On Button"=w1317, "Turn On Indicator"=w1316) -> ("Success?"=w1313:bool)  [unwired: 6 in]
        n676 = Select(t=LongShotStates."Set Digi Mode", s=w1313, f=LongShotStates."Idle") -> (s? t:f=w1314:T13)
      }
      frame "Set Digi Mode" {
        # "Start Digitizer"
        n677 = flat-sequence {
          tunnel: [w1325] -> w1321
          tunnel: w1321 -> [w1330]
          tunnel: [w1330] -> w1320
          tunnel: w1320 -> [w1332]
          frame #0 {
            n678 = control-ref of="Digitizer On"() -> (w1328:refnum<vi>)
            n679 = control-ref of="Start Digi"() -> (w1327:refnum<vi>)
            n680 = call "SwitchTillOn.vi"("Stop if On?"=FALSE, "timeout"=u32 5000, "Turn On Button"=w1327, "Turn On Indicator"=w1328) -> ("Success?"=w1325:bool)  [unwired: 7 in]
          }
          frame #1 {
            n681 = local write "Digi Machine Mode"(DigiMachineStates."Live Mode" ("Digi Machine Mode")) -> ()
          }
          frame #2 {
            n682 = while {
              tunnel: w1332 -> [w1335]
              stop <- w1334 stop-if-true
              n683 = local read "Digi Machine Mode"() -> (w1338:T8)
              n684 = Not(x=w1335) -> (.not. x?=w1333:bool)
              n685 = Equal?(x=w1338, y=DigiMachineStates."Live Mode") -> (x = y?=w1337:bool)
              n686 = Or(x=w1337, y=w1333) -> (x .or. y?=w1334:bool)
            }
          }
        }
      }
      frame "Clear Wave Count" {
        w1339 = TRUE ("Stop Stage")
        n687 = local write "Stop Stage"(w1339) -> ()
        n688 = Select(t=LongShotStates."Set Initial Param", s=w1339, f=LongShotStates."Idle") -> (s? t:f=w1344:T13)
      }
      frame "Set Initial Param" {
        w1347 = u16 512 ("Record Size")
        w1349 = u16 5 items=["1", "2", "4", "8", "16", "32", "64", "128"] ("Amplitude \nAveraging")
        w1346 = u8 2 ("Time Division")
        n689 = Power Of 2(x=w1346) -> (2^x=w1355:dbl)
        n690 = local write "Amplitude \nAveraging"(w1349) -> ()
        n691 = local write "Time Division"(w1346) -> ()
        n692 = local write "Record Size"(w1347) -> ()
        n693 = Divide(x=1600000000.0 ("Sample Rate"), y=w1355) -> (x/y=w1354:dbl)
        n694 = property on="Delay(us)" class="DigNum (strict)"("Val(Sgnl)"=sgl 0.0 ("Delay(us)")) -> ()  [unwired: 2 in, 2 out]
        n695 = Compound Arithmetic op=MULTIPLY(w1354, "Long Shot Time (us)", 1e-06 ("value")) -> (w1352:dbl)
        n696 = Divide(x=w1352, y=w1347) -> (x/y=→"LongShotRunTimes":dbl)
      }
      frame "Set Param" {
        n697 = flat-sequence {
          tunnel: w1362 -> [w1368]
          tunnel: [w1372] -> w1360
          tunnel: w1360 -> [w1378]
          tunnel: [w1377] -> w1359
          frame #0 {
            n698 = local read "Record Size"() -> (w1366:u16)
            n699 = local read "Time Division"() -> (w1370:u8)
            n700 = Power Of 2(x=w1370) -> (2^x=w1371:dbl)
            n701 = Divide(x=w1371, y=1600000000.0 ("Sample Rate")) -> (x/y=w1367:dbl)
            n702 = Compound Arithmetic op=MULTIPLY(w1366, w1367, w1368, u32 1000000 ("value")) -> (w1365:dbl)
            n703 = property on="Delay(us)" class="DigNum (strict)"("Val(Sgnl)"=w1365) -> ()  [unwired: 2 in, 2 out]
          }
          frame #1 {
            n704 = while {
              tunnel: [w1373] -> w1372
              stop <- w1374 stop-if-true
              n705 = local read "Wave out packet"() -> (w1373:T10)
              n706 = local read "Digi State"() -> (w1376:T9)
              n707 = Equal?(x=w1376, y=Digitizer_StatesMain."SetParam") -> (x = y?=w1374:bool)
            }
          }
          frame #2 {
            n708 = Unbundle By Name(w1378) -> ("Wave Count"=w1377:u64)
          }
        }
      }
      frame "Take Shot" {
        w1380 = u64 10  # nth Wave
        # "Taking every 10th Wave After Setting the parameters"
        n709 = local read "Wave out packet"() -> (w1388:T10)
        n710 = Add(x=w1379, y=w1380) -> (x+y=w1381:u64)
        n711 = Unbundle By Name(w1388) -> ("Wave Count"=w1386:u64, "Wave"=w1383:i16[])
        n712 = Greater?(x=w1386, y=w1381) -> (0:w1385:bool)
        n713 = Select(t=LongShotStates."UpdateParam" ("f"), s=w1385, f=LongShotStates."Take Shot") -> (s? t:f=w1387:T13)
      }
      frame "UpdateParam" {
        n714 = local read "LongShotRunTimes"() -> (w1395:u32)
        n715 = Build Array (concatenate)(w1397, w1399) -> (w1398:i16[])
        n716 = Increment(x=w1396) -> (x+1=w1391:u8)
        n717 = Divide(x=w1391, y=w1395) -> (x/y=w1392:dbl)
        n718 = Multiply(x=100.0, y=w1392) -> (x*y=→"ProgressBar\nLongShot":dbl)
        n719 = Less?(x=w1391, y=w1395) -> (x < y?=w1400:bool)
        n720 = Select(t=LongShotStates."Set Param", s=w1400, f=LongShotStates."Show Data") -> (s? t:f=w1403:T13)
      }
      frame "Show Data" {
        n721 = flat-sequence {
          tunnel: w1405 -> [w1413]
          frame #0 {
            n722 = local write "Digi Machine Mode"(DigiMachineStates."Idle Mode" ("Digi Machine Mode")) -> ()
          }
          frame #1 {
            n723 = while {
              stop <- w1410 stop-if-true
              n724 = local read "Digi Machine Mode"() -> (w1411:T8)
              n725 = Equal?(x=w1411, y=DigiMachineStates."Idle Mode") -> (x = y?=w1410:bool)
            }
          }
          frame #2 {
            n726 = local write "Stop Stage"(FALSE ("Stop Stage")) -> ()
            n727 = call "LongShotView.vi"("Data In"=w1413) -> ()  [unwired: 11 in]
          }
        }
      }
    }
    n728 = call <extravilib>:"Read.vi"("channel"=w1292) -> ("element"=w1291:bool)  [unwired: 1 in, 1 out]
  }
  n729 = timed-loop {
    tunnel: w3 -> [w1425]
    timing: w14 -> [_]
    timing-out: [_] -> w13
    tunnel: w12 -> [w1423]
    stop <- w1424 stop-if-true
    n730 = node-c288() -> ()  [unwired: 1 in, 1 out]
    n731 = call <extravilib>:"Read.vi"("channel"=w1423) -> ("element"=w1422:dbl[])  [unwired: 1 in, 1 out]
    n732 = local read "X Step Size (R)"() -> (w1419:sgl)
    n733 = local read "Y Step Size (R)"() -> (w1418:sgl)
    n734 = local read "Line Count"() -> (w1426:u64)
    n735 = local read "Pixel Count"() -> (w1427:u64)
    n736 = property on="Image Display" class="IntGraph (strict)"("XScale.Multiplier"=w1419, "YScale.Multiplier"=w1418) -> ()  [unwired: 2 in, 2 out]
    n737 = Reshape Array(w1422, w1426, w1427) -> (w1421:dbl[][])
    n738 = call "Rotate Array 2012 NIVerified.vi"("Rotation CW/nCCW"=TRUE ("Rotation \nOrientation"), "Rotation"=enum8{"90", "180", "270"}."90", "Array"=w1421) -> ("Rotated 2D Array"=→"Image Display":dbl[][])  [unwired: 8 in]
    n739 = call <extravilib>:"Read.vi"("channel"=w1425) -> ("element"=w1424:bool)  [unwired: 1 in, 1 out]
    n740 = call "IntensityColorTables.vi"("Map Selector"="Colormap Selector") -> ("Color Map Array"=w1416:u32[])  [unwired: 10 in]
    n741 = property on="Image Display" class="IntGraph (strict)"("Color Table"=w1416) -> ()  [unwired: 2 in, 2 out]
    n742 = node-c288() -> ()  [unwired: 1 in, 1 out]
  }
  n743 = node-c288(w13) -> ()  [unwired: 1 out]
  n744 = node-c288(w63) -> ()  [unwired: 1 out]
  n745 = disable-structure shown="Disabled" {
    frame Disabled {
      n746 = control-ref of="Scanned Image"() -> ()  [unwired: 1 out]
      n747 = call "DisplayImagePlot.vi"("Colorbar"="ColorBar", "Axis"="Axis", "Map"="Map") -> ("Picture"=→"Scanned Image":picture, "Data Array"=w1435:dbl[][], "Picture For Size Ref"=w1434:refnum<vi>)  [unwired: 6 in]
      n748 = call <vilib>:"create_plot_surface.vi"() -> ("plots out"=→"Topography Plot":refnum<class "Base Datatype.lvclass">[], "z matrix"=w1438:dbl[][])  [unwired: 4 in, 6 out]
      n749 = property on="Topography Plot" class="LabVIEW 3D Graph (strict)"("property_graph_fast_draw"=TRUE ("Graph:Fast Draw")) -> ()  [unwired: 2 in, 2 out]
    }
    frame Enabled {
    }
  }
  n750 = node-c288(w1) -> ()  [unwired: 1 out]
